vi "XY_plot_gnuplot.vi"(0 "Plot Array":cluster{dbl[], dbl[]}[](array[cluster])=[{[500.0, 500.0, 953.54, 215.0, 270.0, 320.0, 445.0, 525.0, 600.0, 675.0, 750.0, 825.0, 900.0, 960.0, 1010.0, 1060.0], [4.614524, 4.54365, 5.818368, 0.1374656, 0.6662545, 1.465458, 3.619824, 4.848976, 5.887329, 5.940571, 6.152151, 5.717487, 5.600293, 5.40069, 5.154843, 5.121789]}, {[100.0, 150.0, 215.0, 270.0, 320.0, 445.0, 525.0, 600.0, 675.0, 750.0, 825.0, 900.0, 960.0, 1010.0, 1060.0], [0.002314715, -0.00693192, 0.120417, 0.6880509, 1.519176, 3.513709, 5.065183, 6.116033, 6.096773, 5.938465, 5.593788, 5.5597, 5.387002, 5.304077, 4.887903]}] {"?" format="%.2f"; "?" format="%.2f"}, 1 "Job Directory":path=path "/G4_2_HD/Users/paulhayden/Documents/Projects/Westlakes_resolution") -> (2 "Saved Automatically?":bool, 3 "Tex Info String":string="set term epslatex\nset output \"Plot.eps\"\nset xlabel '$Distance~(m)$'\nset ylabel '$DF~(s/m^3)\\times10^6$'\nset samples 1000\nset pointsize 1.00\nset title '$B38~Centreline~Glc$' 0, 0\nset size 0.75,0.9\n\n#set key 450, -2.5833\n unset key\nset label 1 '~~~~~~~~~~~Angle~(deg)~=~0' at -100, -2.58\nset label 2 '~~~~~~~~~~~Height~(m)~=~5' at -100, -3.27\n set xrange [0 : 500] \n# set autoscale x \n set yrange [0.10000 : 7]\n# set autoscale y \n\nplot \"B38_Centreline_Glc.dat\" index 0 using 1:2 axes x1y1 title '$File=B38R~DDD.xls$' with points 1 1, \\\n\"B38_Centreline_Glc.dat\" index 1 using 1:2 axes x1y1 title '$File=B38R~DDD~1.xls$' with points 1 3", 4 "Plot data file":path)   [LabVIEW 2014]
uses:
  Gnuplot_Label.ctl
  gnuplotScriptComponents/gridlines.ctl
  gnuplotScriptComponents/legendProperties.ctl
  gnuplotScriptComponents/legendAppearance.ctl
  gnuplotScriptComponents/alignment.ctl
  gnuplotScriptComponents/at.ctl
  <vilib>/Analysis/baseanly.llb/Mean (DBL).vi
  Results_plotter_Global.vi
  <vilib>/Analysis/NI_AALBase.lvlib
  <vilib>/Analysis/NI_AALPro.lvlib
panel:
  in  "Show Re-Run Gnuplot?":bool
  in  "Tab Control":T1(tab)
  in  "Plot Title":u16(ring) items=["Title String Only", "Project::", "Case2::", "Case::", "Date::", "File::", "Ref Velocity:(m/s):", "Source:Location:X (mm)", "Source:Location:Y (mm)", "Source:Location:Z (mm)", "Source:Internal Diameter:(mm)", "Model:Orientation:", "Carrier:Gas:", "Trace:Gas:", "Q:Source:(l/min)", "Q:Trace:(l/min)", "Source:Density:Ratio", "Source::", "X (mm)::", "Y (mm)::", "Z(mm)::", "Location:XY:", "Location:XZ:", "Profiles::", "U/U(ref)::", "V/U(ref)::", "W/U(ref)::", "u^2/U_{ref}^2::", "v^2/U_{ref}^2::", "w^2/U_{ref}^2::", "uv/U_{ref}^2::", "-uw/U_{ref}^2::", "CU(ref)/Q::(m^{-2})", "c'U(ref)/Q::(m^{-2})", "uc/Q::(m^{-2})", "vc/Q::(m^{-2})", "wc/Q::(m^{-2})", "Measurement:Time:(min)", "U::(m/s)", "U:(m/s):St Error", "V::(m/s)", "W::(m/s)", "W:(m/s):St Error", "u^2::(m/s)^2", "v^2::(m/s)^2", "w^2::(m/s)^2", "uv::(m/s)^2", "uw::(m/s)^2", "C:Trace:(ppm)", "C:Trace (ppm):St Error", "c^2::(ppm)^2", "uc::(ppm m/s)", "vc::(ppm m/s)", "wc::(ppm m/s)", "u^2:(m/s)^2:St Error", "w^2:(m/s)^2:St Error", "U/U(ref)::St Error", "W/U(ref)::St Error", "u^2/U_{ref}^2::St Error", "w^2/U_{ref}^2::St Error", "Raw:Data:Filename", "EnFlo_Tunnel:Inlet_Temp:St Deviation", "Instrumentation::", "Number of:FFID Samples:per Block", "Total Number:of FFID Spikes:Removed", "LDA (U):Timescale Estimate:Integrated to 25%", "Number Of:Measurement:Blocks", "LDA:Sampling Rate:(Hz)", "Number of:LDA Samples:per Block", "Multi Run:Start Time:", "Bkgnd:FF (C):", "Bkgnd Variance:FF (C):", "Seconds:since:1st Jan", "Drift%::", "CU/Q::Err", "EnFlo Lab:labstrat1:Delta T", "GMU:Carrier 2:Gas", "Emission:Velocity:m/s", "Emission:Ratio:", "FF (C):Standard Error:in Variance", "GMU:Source:Type", "Aero_Tunnel:Speed:Meas Velocity", "Multi Run:Row:Number", "EnFlo_Tunnel:FFID:Temp", "FF (C):Calibration:Filename", "Source2:Enable:", "GMU:Source:Dem Q", "Multi Run:Command:Filename", "Thermistor:Temp:", "University:Outside:Temp", "Spires::", "Run::", "Roughness::", "Dem_Uref::", "Comments::", "X:Tunnel:(mm)", "EnFlo_Tunnel:Trav Origin:X Offset", "Run_::", "EnFlo_Tunnel Metadata:Source:Number", "EnFlo_Tunnel Metadata:Model:Trees", "w'::", "EnFlo_Stack:Floor:Surface (mm)", "Z (mm)::Raw", "EnFlo_Tunnel:Shaft:rpm", "u'/U::", "EnFlo_Tunnel:Trav1 Pos:X", "EnFlo_Tunnel:Inlet:K_Factor", "EnFlo_Tunnel:Inlet_Temp:Average", "Number of Measurements"]
  in  "Plot Title":string
  in  "Added labels":i32[](listbox)
  in  "Show Labels?":bool
  in  "Summarise":u16(ring) items=["All Series", "X (mm)=-910__Z(mm)=35__"]
  in  "X Log?":bool
  in  "Y Log?":bool
  in  "Ymin Val":dbl
  in  "Ymin":bool=TRUE
  in  "Xmin Val":dbl
  in  "Xmin":bool=TRUE
  in  "Xmax Val":dbl
  in  "Xmax":bool=TRUE
  in  "Ymax Val":dbl
  in  "Ymax":bool=TRUE
  in  "Major Gridlines":T2
  in  "Minor Gridlines":T2
  out "Time format?":bool
  in  "precision":string
  out "Profile offset":dbl
  in  "Offset?":bool
  in  "Mode":T3
  in  "Separation":dbl=1.2
  in  "Fit Line Width":i32=2
  in  "Fit type":T4(ring)
  in  "Put Coeff\nin Results file":bool
  in  "Analysis":T5(ring)
  in  "Wavelength?":bool
  in  "Auto Zp":bool=TRUE
  in  "Fixed Zp":dbl format="%.2f"
  in  "Something about fit..!":bool
  in  "Fit Line Type":i32=2
  in  "Black and white?":bool
  in  "plot error bars?":bool
  in  "Plot style":u16[](array[ring])=[0, 0, 0, 0, 0, 0, 0, 0, 0, 0, 0] items=["points", "lines", "linespoints"]
  in  "Point Size":dbl=1.2 format="%.2f"
  in  "Graph Height":string="0.9"
  in  "Graph width":string="0.75"
  in  "Show legend?":bool
  in  "Legend Position":u16(ring) items=["LabVIEW calculated", "top left", "top right", "bottom left", "bottom right", "below"]
  in  "Reverse order":bool
  in  "Save data analysis file":bool
  out "Path":path
  in  "Filename Max length":i32=28
  out "With legend":i32=580
  out "No Legend":i32=397
  out "No of Series":i32=2
  out "X location":dbl=-100.0
  out "Y location":dbl=-2.583333333333333
  out "Delta y":dbl=0.6900000000000001
  out "Extra range":dbl
  out "Final Title":string="B38 Centreline Glc"
  out "XY Graph":cluster{dbl[], dbl[]}[](graph)=[{[215.0, 270.0, 320.0, 445.0, 500.0, 500.0, 525.0, 600.0, 675.0, 750.0, 825.0, 900.0, 953.54, 960.0, 1010.0, 1060.0], [0.1374656, 0.6662545, 1.465458, 3.619824, 4.614524, 4.54365, 4.848976, 5.887329, 5.940571, 6.152151, 5.717487, 5.600293, 5.818368, 5.40069, 5.154843, 5.121789]}, {[100.0, 150.0, 215.0, 270.0, 320.0, 445.0, 525.0, 600.0, 675.0, 750.0, 825.0, 900.0, 960.0, 1010.0, 1060.0], [0.002314715, -0.00693192, 0.120417, 0.6880509, 1.519176, 3.513709, 5.065183, 6.116033, 6.096773, 5.938465, 5.593788, 5.5597, 5.387002, 5.304077, 4.887903]}]
  # "Scales"
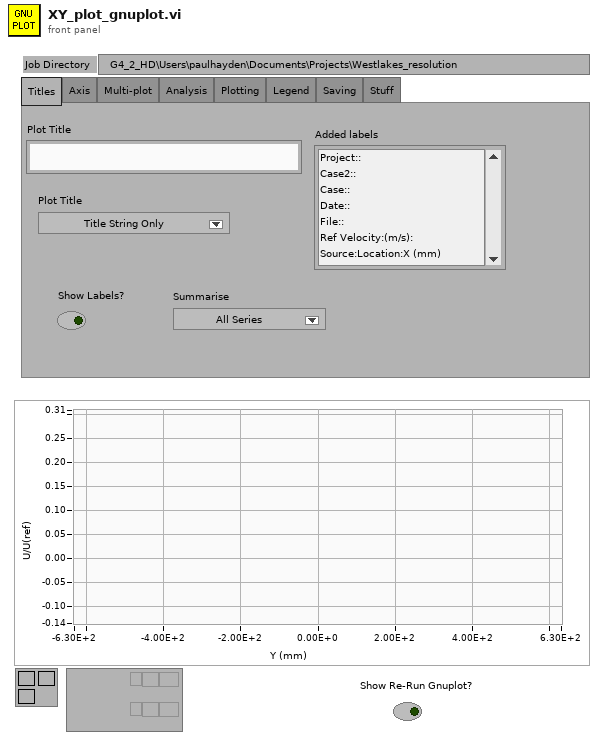
[diagram p1: front panel]
types:
  T1 = enum32{"Titles", "Axis", "Multi-plot", "Analysis", "Plotting", "Legend", "Saving", "Stuff"}
  T2 = typedef "gridlines.ctl" = enum16{"None", "X only", "Y only", "Both X and Y"}
  T3 = typedef "Gnuplot_Label.ctl" = enum16{"3 Labels per plot", "Only Center label", "Only Bottom Label"}
  T4 = enum16{"None", "Spline", "Linear", "2nd Poly", "3rd Poly", "4th Poly", "Gauss Lat", "Gauss vert", "Gauss Vert with 2 sig", "Guass glc"}
  T5 = enum16{"None", "% change", "Spectrum", "Norm Spec"}
  T6 = cluster{"Output":dbl[], "PercentageDifferenceArray":dbl[]}[]
  T7 = cluster{"Output":dbl[], "PercentageDifferenceArray":dbl[]}
  T8 = typedef "legendProperties.ctl" = cluster{"Appearance":T9, "Alignment":T10, "Location":string, "\"At\" location":T11}
  T9 = typedef "legendAppearance.ctl" = cluster{"layout":string, "text-sample order":string, "key order":string, "surroundingBox":string, "MaxRows":u32, "MaxCols":u32, "WidthAdjust":dbl}
  T10 = typedef "alignment.ctl" = cluster{"Horizontal":string, "Vertical":string}
  T11 = typedef "at.ctl" = cluster{"XcoordSys":string, "YcoordSys":string, "Xvalue":dbl, "Yvalue":dbl}
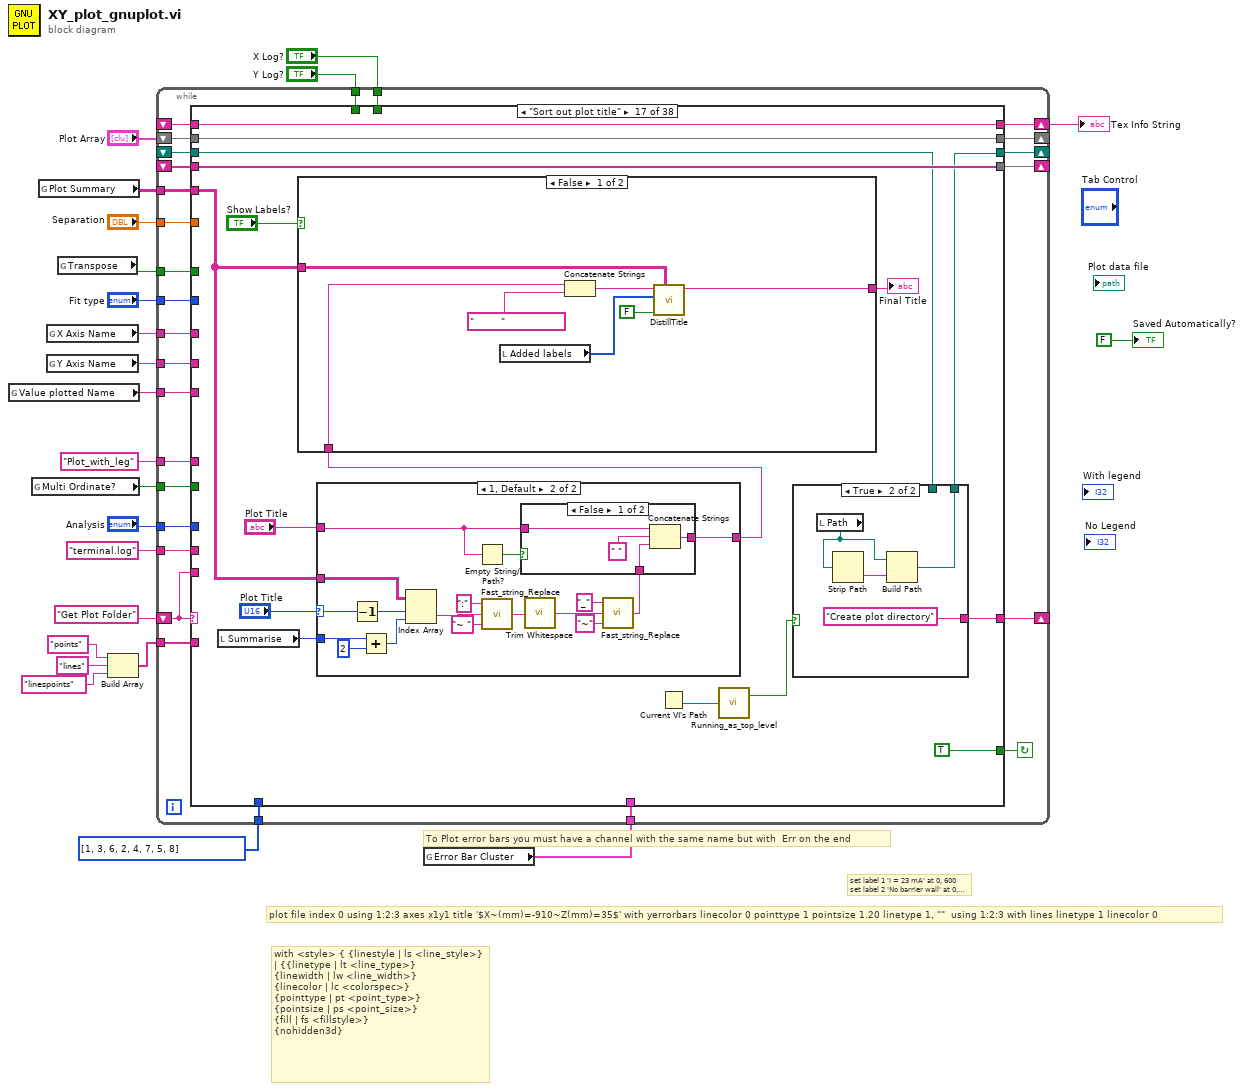
[diagram p0: block diagram]
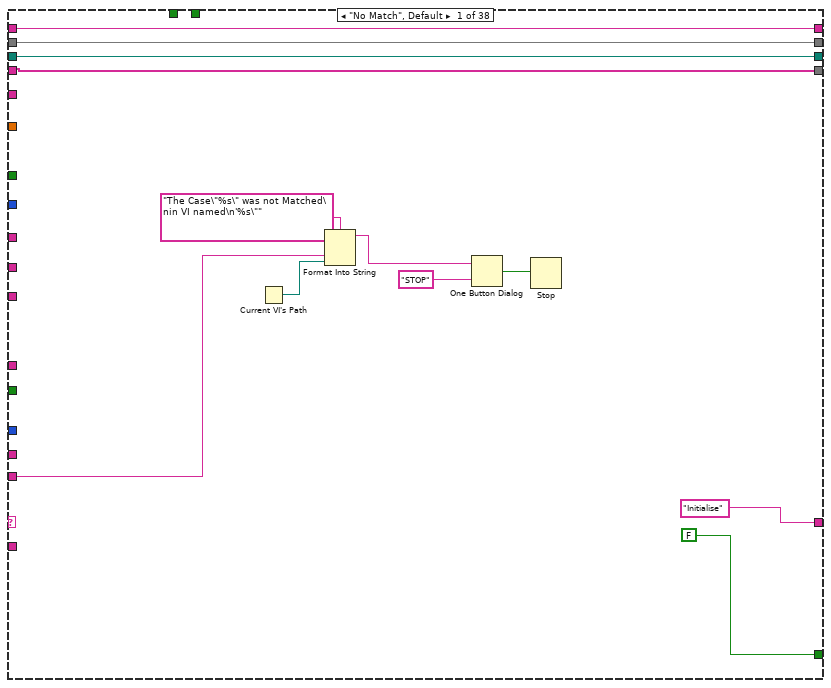
[diagram p2: hidden frame]
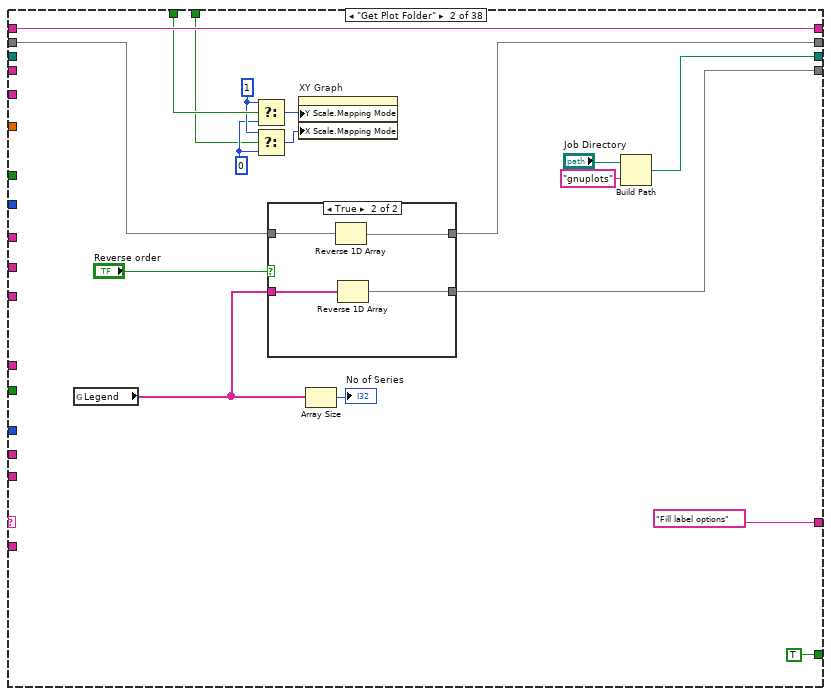
[diagram p3: hidden frame]
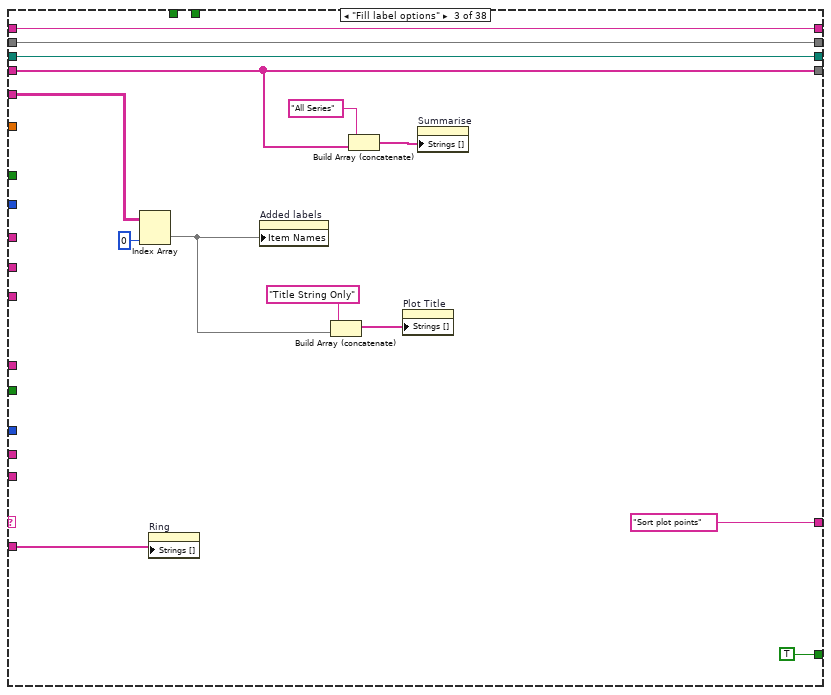
[diagram p5: hidden frame]
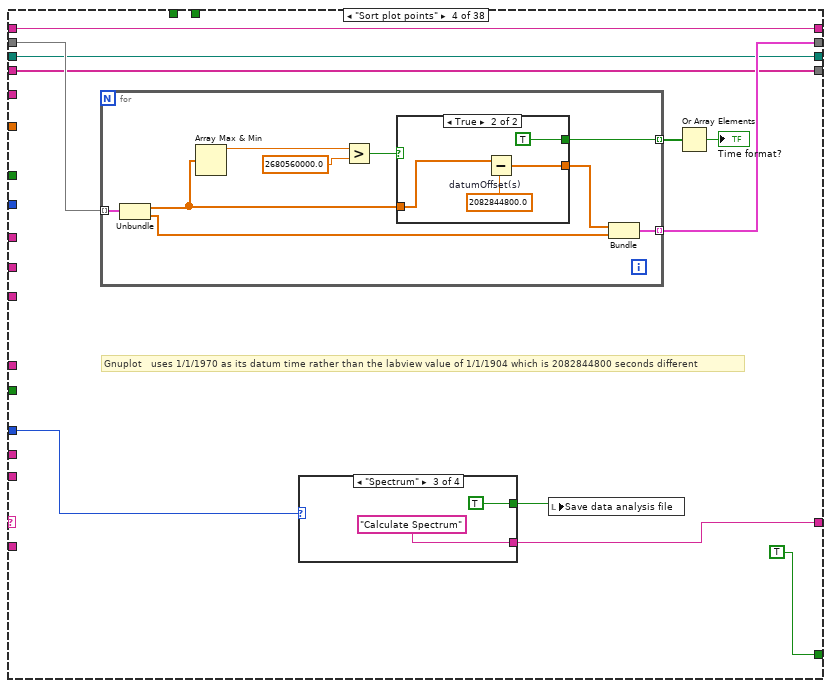
[diagram p6: hidden frame]
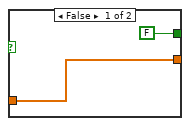
[diagram p7: hidden frame]
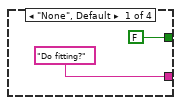
[diagram p8: hidden frame]
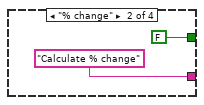
[diagram p9: hidden frame]
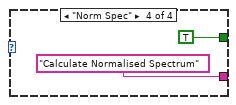
[diagram p10: hidden frame]
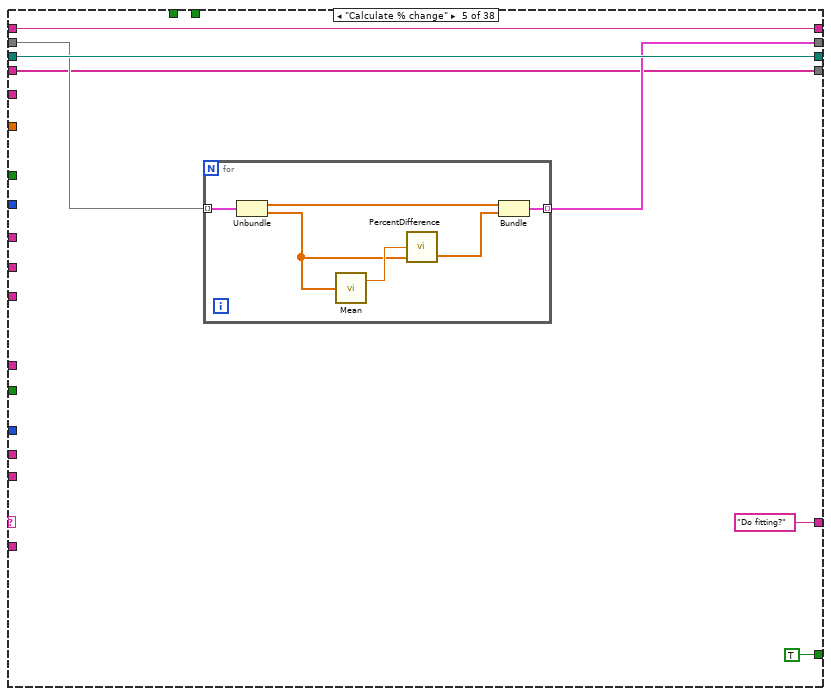
[diagram p11: hidden frame]
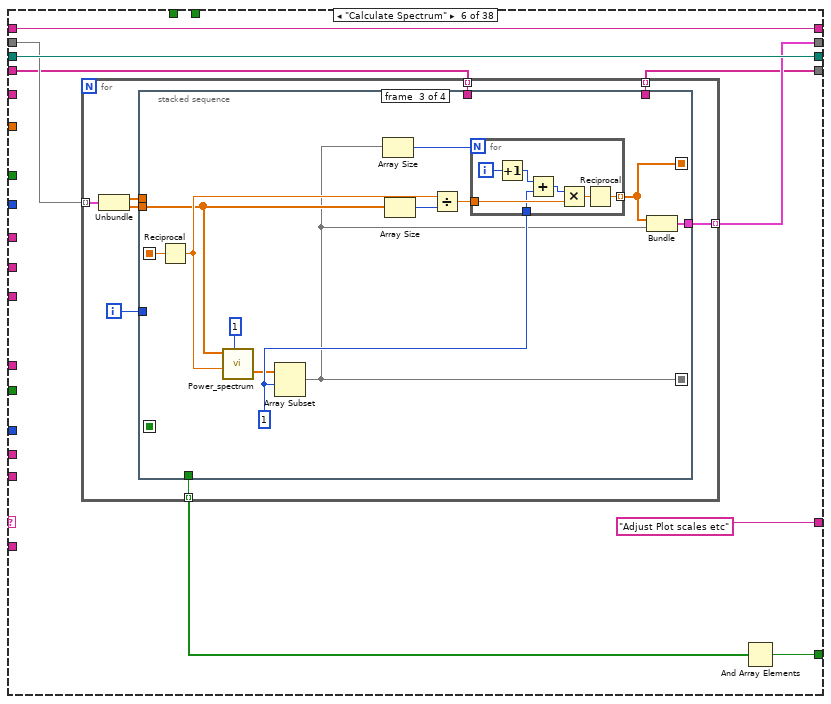
[diagram p12: hidden frame]
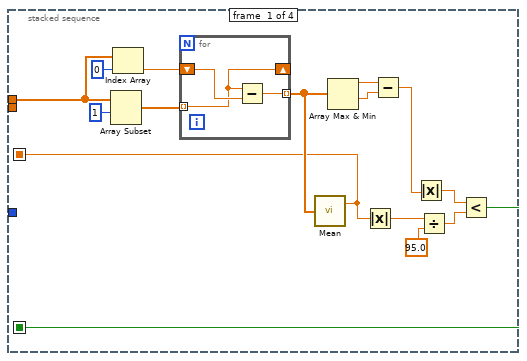
[diagram p13: hidden frame]
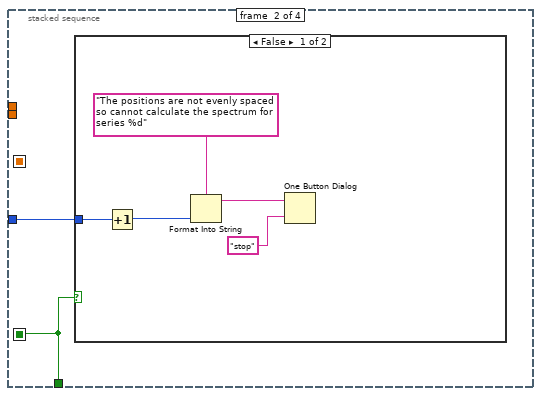
[diagram p14: hidden frame]
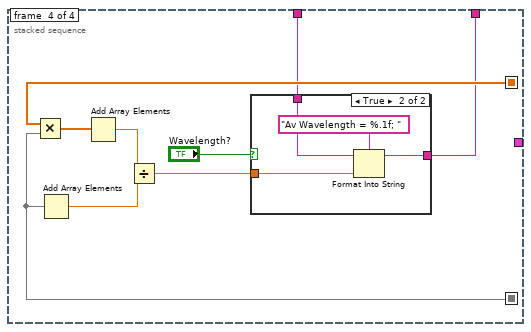
[diagram p16: hidden frame]
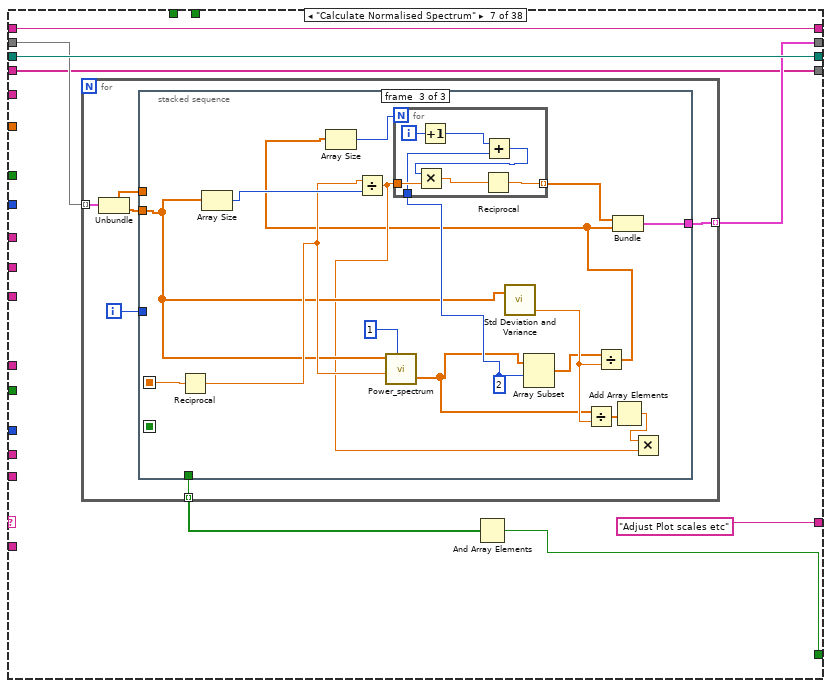
[diagram p18: hidden frame]
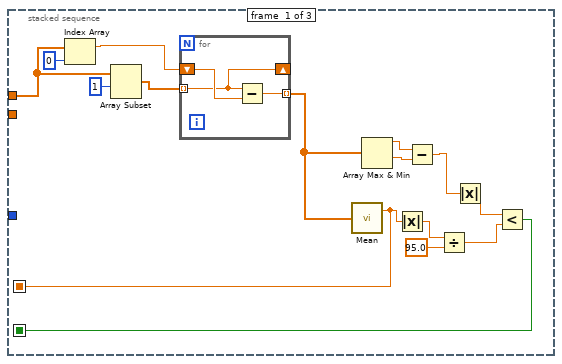
[diagram p19: hidden frame]
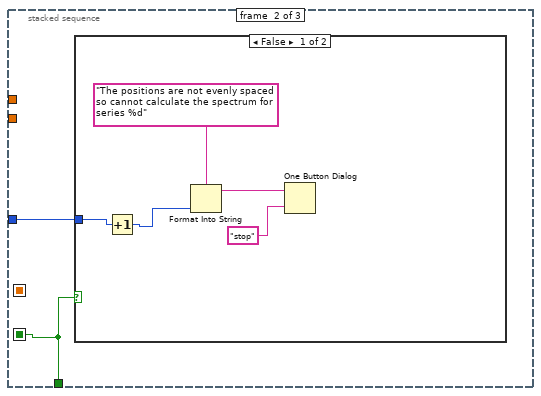
[diagram p20: hidden frame]
diagram:
  # "plot file index 0 using 1:2:3 axes x1y1 title '$X~(mm)=-910~Z(mm)=35$' with yerrorbars linecolor 0 pointtype 1 pointsize 1.20 linetype 1, \"\"  using 1:2:3 with lines linetype 1 linecolor 0"
  # "with <style> { {linestyle | ls <line_style>} \n| {{linetype | lt <line_type>} \n{linewidth | lw <line_width>} \n{linecolor | lc <colorspec>} \n{pointtype | pt <point_type>} \n{pointsize | ps <point_size>} \n{fill | fs <fillstyle>} \n{nohidden3d}"
  # "To Plot error bars you must have a channel with the same name but with  Err on the end"
  # "set label 1 'I = 23 mA' at 0, 600\nset label 2 'No barrier wall' at 0, 300"
  n1 = global read "Results_plotter_Global.vi" "Value plotted Name"() -> (w19:string)
  n2 = global read "Results_plotter_Global.vi" "Multi Ordinate?"() -> (w1:bool)
  n3 = global read "Results_plotter_Global.vi" "Plot Summary"() -> (w22:string[][])
  n4 = global read "Results_plotter_Global.vi" "X Axis Name"() -> (w21:string)
  n5 = global read "Results_plotter_Global.vi" "Y Axis Name"() -> (w20:string)
  n6 = global read "Results_plotter_Global.vi" "Transpose"() -> (w2:bool)
  n7 = Build Array("points", "lines", "linespoints") -> (w9:string[])
  n8 = global read "Results_plotter_Global.vi" "Error Bar Cluster"() -> (w4:cluster{string[]}[])
  n9 = while {
    shift-left: "Get Plot Folder" -> [w48]
    shift-right: [w49] -> _
    tunnel: w22 -> [w47]
    shift-right: [w46] -> _
    shift-left: _ -> [w45]
    tunnel: "Analysis" -> [w44]
    tunnel: w21 -> [w43]
    tunnel: w20 -> [w42]
    tunnel: w19 -> [w41]
    shift-right: [w39] -> _
    shift-left: "Plot Array" -> [w40]
    shift-right: [w37] -> w17
    shift-left: _ -> [w38]
    tunnel: "Plot_with_leg" ("name or relative path") -> [w36]
    tunnel: "Fit type" -> [w35]
    shift-right: [w34] -> _
    shift-left: _ -> [w33]
    tunnel: "terminal.log" -> [w32]
    tunnel: w9 -> [w31]
    tunnel: i32[] [1, 3, 6, 2, 4, 7, 5, 8] ("Plot style") -> [w30]
    tunnel: "Separation" -> [w29]
    tunnel: "Y Log?" -> [w28]
    tunnel: w4 -> [w27]
    tunnel: "X Log?" -> [w26]
    tunnel: w2 -> [w25]
    tunnel: w1 -> [w24]
    stop <- w50 continue-if-true
    n10 = case shown="\"Sort out plot title\"" w48 {
      tunnel: [FALSE TRUE TRUE ("Top Level") TRUE TRUE w150 w223 TRUE TRUE TRUE ("Top Level") TRUE ("Top Level") TRUE ("Top Level") TRUE ("Top Level") TRUE ("Top Level") TRUE ("Top Level") TRUE ("Top Level") TRUE ("Top Level") TRUE ("Top Level") TRUE ("Top Level") TRUE ("Top Level") w674 w747 TRUE ("Top Level") TRUE ("Top Level") TRUE ("Top Level") TRUE ("Top Level") TRUE ("Top Level") TRUE ("Top Level") TRUE ("Top Level") TRUE ("Top Level") TRUE ("Top Level") TRUE ("Top Level") TRUE ("Top Level") TRUE ("Top Level") TRUE ("Top Level") w1570 FALSE ("Top Level") FALSE ("Top Level")] -> w50
      tunnel: ["Initialise" "Fill label options" "Sort plot points" w104 "Do fitting?" "Adjust Plot scales etc" "Adjust Plot scales etc" "Adjust Plot scales etc" "Add fitted line styles" "Adjust Plot scales etc" w381 "Fill Second legend" "Fill Second legend" "Fill Second legend" "Calculate plot max and min values" "Sort out plot title" w566 w636 "Create plot directory" w660 w673 w746 w890 "Edit Legend names" w1074 "Labels?" ("t") "Labels?" ("t") w1235 w1246 "Plot Command" "Write gnuplot file" ("t") "Execute shell script" ("t") "Has pdf been generated?" ("t") w1546 "Input Fit Coefficients into results file?" "Read Fit Coefficients" ("t") "End" ("t") "End" ("t")] -> w49
      tunnel: w48 -> [w57 _ _ _ _ _ _ _ _ _ _ _ _ _ _ _ _ _ _ _ _ _ _ _ _ _ _ _ _ _ _ _ _ _ _ _ _ _]
      tunnel: w47 -> [_ _ w100 _ _ _ _ _ _ _ _ _ _ _ _ _ w575 _ _ _ w672 w745 _ _ _ _ _ _ w1245 _ _ _ _ _ _ _ _ _]
      tunnel: [w54 w77 w94 w108 w139 w155 w229 w290 w305 w366 w391 w417 w426 w438 w465 w499 w568 w637 w648 w662 w675 w748 w902 w942 w1089 w1156 w1212 w1242 w1252 w1376 w1408 w1531 w1539 w1552 w1563 w1574 w1592 w1679] -> w46
      tunnel: w45 -> [w54 _ w94 w108 w139 w155 w229 w290 w305 w366 w391 w417 w426 w438 w461 w499 w567 w633 w649 w657 w675 w748 w902 w942 w1089 w1156 w1212 w1242 w1252 w1376 w1408 w1531 w1539 w1552 w1563 w1574 w1592 w1679]
      tunnel: w44 -> [_ _ _ w105 _ _ _ _ _ _ w382 _ _ w432 _ _ _ w624 _ _ w668 w740 w899 _ _ _ _ _ _ _ _ _ _ _ _ _ _ _]
      tunnel: w43 -> [_ _ _ _ _ _ _ _ w296 _ _ w413 w425 _ _ _ _ _ _ _ w671 w744 w897 _ _ _ _ _ _ _ _ _ _ _ _ _ _ _]
      tunnel: w42 -> [_ _ _ _ _ _ _ _ w295 _ _ w412 w424 w437 _ _ _ _ _ _ w670 w743 w898 _ _ _ _ _ _ _ _ _ _ _ _ _ _ _]
      tunnel: w41 -> [_ _ _ _ _ _ _ _ _ _ _ _ _ _ _ _ _ _ _ _ w667 _ _ _ _ _ _ _ _ _ _ _ _ _ _ _ w1586 _]
      tunnel: w40 -> [w53 w72 w95 w110 w138 w154 w228 w286 w301 w365 w380 w416 w423 w436 w464 w496 w581 w635 w652 w665 w666 w742 w903 w929 w1084 w1151 w1208 w1239 w1247 w1377 w1409 w1537 w1544 w1559 w1568 w1578 w1581 w1684]
      tunnel: [w53 w71 w95 w109 w137 w153 w227 w286 w294 w365 w380 w416 w423 w436 w464 w496 w581 w635 w652 w665 w666 w739 w903 w929 w1084 w1151 w1208 w1239 w1247 w1377 w1409 w1537 w1544 w1559 w1568 w1578 w1581 w1684] -> w39
      tunnel: w38 -> [w52 w76 w96 w107 w136 w152 w226 w289 w304 w363 w383 w415 w422 w435 w463 w500 w576 w634 w651 w664 w676 w749 _ w940 w1088 w1122 w1188 w1230 w1249 w1373 w1406 w1526 w1542 w1557 w1566 w1576 w1595 w1682]
      tunnel: [w52 w76 w96 w107 w136 w152 w226 w289 w304 w363 w383 w415 w422 w435 w463 w500 w576 w634 w651 w664 w676 w749 w893 w938 w1088 w1119 w1187 w1229 w1250 w1369 w1405 w1526 w1542 w1557 w1566 w1576 w1595 w1682] -> w37
      tunnel: w36 -> [_ _ _ _ _ _ _ _ _ _ _ _ _ _ _ _ _ _ _ _ _ _ _ _ _ _ _ _ _ _ _ _ _ _ _ _ _ _]
      tunnel: w35 -> [_ _ _ _ _ _ _ w287 w303 _ w385 _ _ _ _ _ _ _ _ _ _ _ w891 w944 _ _ _ _ _ w1342 w1402 _ _ _ _ w1573 w1588 _]
      tunnel: [w51 w70 w92 w106 w135 w148 w225 w288 w298 w362 w387 w414 w421 w434 w462 w498 w580 w632 w650 w663 w669 w741 w901 w945 w1090 w1155 w1211 w1241 w1251 w1363 w1407 w1532 w1543 w1558 w1567 w1577 w1596 w1683] -> w34
      tunnel: w33 -> [w51 _ w92 w106 w135 w149 w225 w288 w299 w362 w387 w414 w421 w434 w462 w498 w580 w632 w650 w663 w669 w741 w901 w945 w1091 w1155 w1211 w1241 w1251 w1363 w1407 w1532 w1543 w1558 w1567 w1577 w1596 w1683]
      tunnel: w32 -> [_ _ _ _ _ _ _ _ _ _ _ _ _ _ _ _ _ _ _ _ _ _ _ _ _ _ _ _ _ _ _ _ w1538 _ _ _ _ w1677]
      tunnel: w31 -> [_ _ w90 _ _ _ _ _ _ _ _ _ _ _ _ _ _ _ _ _ _ _ _ _ _ _ _ _ _ _ _ _ _ _ _ _ _ _]
      tunnel: w30 -> [_ _ _ _ _ _ _ _ _ _ _ _ _ _ _ _ _ _ _ _ _ _ _ _ _ _ _ _ _ _ w1400 w1528 _ _ _ _ _ _]
      tunnel: w29 -> [_ _ _ _ _ _ _ _ _ _ _ _ _ _ _ _ _ _ _ _ _ w738 _ _ w1083 _ _ _ _ w1360 _ _ _ _ _ _ _ _]
      tunnel: w28 -> [_ w69 _ _ _ _ _ _ _ _ _ _ _ _ _ _ _ _ _ _ _ _ _ _ _ w1135 w1199 _ w1244 w1357 _ _ _ _ _ _ _ _]
      tunnel: w27 -> [_ _ _ _ _ _ _ _ _ _ _ _ _ _ _ w469 _ _ _ _ _ w737 _ _ _ _ _ _ _ _ w1399 _ _ _ _ _ _ _]
      tunnel: w26 -> [_ w64 _ _ _ _ _ _ _ _ _ _ _ _ _ _ _ _ _ _ _ _ _ _ _ w1132 _ _ w1243 w1352 _ _ _ _ _ _ _ _]
      tunnel: w25 -> [_ _ _ _ _ _ _ _ _ _ _ _ _ _ _ w467 _ _ _ _ _ w736 _ w930 _ _ _ _ _ w1347 w1396 _ _ _ _ _ _ _]
      tunnel: w24 -> [_ _ _ _ _ _ _ _ _ _ _ _ _ _ _ _ _ _ _ _ _ _ _ _ _ _ _ _ _ _ _ _ _ _ _ _ _ _]
      frame "No Match", Default {
        n11 = Current VI's Path() -> (path=w56:path)
        n12 = Format Into String(format string="The Case\"%s\" was not Matched\nin VI named\n'%s\"" ("Format String"), w57, w56) -> (resulting string=w60:string)  [unwired: 2 in, 1 out]
        n13 = One Button Dialog(message=w60, button name ("OK")="STOP") -> (true=w58:bool)
        n14 = Stop(stop? (T)=w58) -> ()
      }
      frame "Get Plot Folder" {
        w65 = u8 0 ("f")
        w66 = u8 1 ("Y Scale.Mapping Mode")
        n15 = global read "Results_plotter_Global.vi" "Legend"() -> (w63:string[])
        n16 = Select(t=w66, s=w69, f=w65) -> (s? t:f=w68:u8)
        n17 = Select(t=w66, s=w64, f=w65) -> (s? t:f=w67:u8)
        n18 = case shown="True" "Reverse order" {
          tunnel: w72 -> [w82 w86]
          tunnel: [w82 w85] -> w71
          tunnel: w63 -> [w81 w84]
          tunnel: [w81 w83] -> w70
          frame False {
          }
          frame True {
            n19 = Reverse 1D Array(array=w86) -> (reversed array=w85:T6)
            n20 = Reverse 1D Array(array=w84) -> (reversed array=w83:string[])
          }
        }
        n21 = property on="XY Graph" class="XYGraph (strict)"("Y Scale.Mapping Mode"=w68, "X Scale.Mapping Mode"=w67) -> ()  [unwired: 2 in, 2 out]
        n22 = Array Size(array=w63) -> (size(s)=→"No of Series":i32)
        n23 = Build Path(base path="Job Directory", name or relative path="gnuplots") -> (appended path=w77:path)
      }
      frame "Fill label options" {
        n24 = Index Array(array=w100, index (col)=0 ("disabled index (col)")) -> (element=w88:string[])  [unwired: 1 in]
        n25 = property on="Ring" class="Ring (strict)"("Strings []"=w90) -> ()  [unwired: 2 in, 2 out]
        n26 = property on="Added labels" class="LstBox (strict)"("Item Names"=w88) -> ()  [unwired: 2 in, 2 out]
        n27 = Build Array (concatenate)("Title String Only", w88) -> (w87:string[])
        n28 = Build Array (concatenate)("All Series", w92) -> (w93:string[])
        n29 = property on="Plot Title" class="Ring (strict)"("Strings []"=w87) -> ()  [unwired: 2 in, 2 out]
        n30 = property on="Summarise" class="Ring (strict)"("Strings []"=w93) -> ()  [unwired: 2 in, 2 out]
      }
      frame "Sort plot points" {
        # "Gnuplot   uses 1/1/1970 as its datum time rather than the labview value of 1/1/1904 which is 2082844800 seconds different"
        n31 = for {
          tunnel: w110 -> [w119] mode=indexing
          tunnel: [w120] -> w109 mode=indexing
          tunnel: [w112] -> w102 mode=indexing
          n32 = Unbundle(w119) -> ("Output"=w115:dbl[], "PercentageDifferenceArray"=w116:dbl[])
          n33 = Array Max & Min(array=w115) -> (max value=w118:dbl)  [unwired: 3 out]
          n34 = Greater?(x=w118, y=2680560000.0) -> (0:w113:bool)
          n35 = case shown="True" w113 {
            tunnel: w115 -> [w122 w126]
            tunnel: [w122 w124] -> w114
            tunnel: [FALSE TRUE] -> w112
            frame False {
            }
            frame True {
              w125 = 2082844800.0  # datumOffset(s)
              n36 = Subtract(x=w126, y=w125) -> (x-y=w124:dbl[])
            }
          }
          n37 = Bundle("Output"=w114, "PercentageDifferenceArray"=w116) -> (w120:T7)  [unwired: 1 out]
        }
        n38 = case shown="\"Spectrum\"" w105 {
          tunnel: ["Do fitting?" "Calculate % change" "Calculate Spectrum" "Calculate Normalised Spectrum"] -> w104
          tunnel: [FALSE ("Save data analysis file") FALSE ("Save data analysis file") TRUE ("Save data analysis file") TRUE ("Save data analysis file")] -> w103
          frame "None", Default {
          }
          frame "% change" {
          }
          frame "Spectrum" {
          }
          frame "Norm Spec" {
          }
        }
        n39 = local write "Save data analysis file"(w103) -> ()
        n40 = Or Array Elements(Boolean array=w102) -> (logical OR=→"Time format?":bool)
      }
      frame "Calculate % change" {
        n41 = for {
          tunnel: w138 -> [w147] mode=indexing
          tunnel: [w145] -> w137 mode=indexing
          n42 = Unbundle(w147) -> ("Output"=w146:dbl[], "PercentageDifferenceArray"=w143:dbl[])
          n43 = call-poly <vilib>:"Mean.vi"("X"=w143) -> ("mean"=w144:dbl)  [unwired: 1 out]
          n44 = call "PercentDifference.vi"("CompareeArray"=w143, "Basis"=w144) -> ("PercentageDifferenceArray"=w142:dbl[])  [unwired: 1 in, 1 out]
          n45 = Bundle("Output"=w146, "PercentageDifferenceArray"=w142) -> (w145:T7)  [unwired: 1 out]
        }
      }
      frame "Calculate Spectrum" {
        n46 = for {
          tunnel: w154 -> [w163] mode=indexing
          tunnel: [w164] -> w153 mode=indexing
          tunnel: [w159] -> w151 mode=indexing
          tunnel: w149 -> [w158] mode=indexing
          tunnel: [w157] -> w148 mode=indexing
          i -> [w160]
          n47 = Unbundle(w163) -> ("Output"=w161:dbl[], "PercentageDifferenceArray"=w162:dbl[])
          n48 = stacked-sequence {
            seq-local: [w166 _ _ _] -> [_ _ w196 _]
            seq-local: [w165 _ _ _] -> [_ w183 _ _]
            seq-local: [_ _ w191 _] -> [_ _ _ w216]
            seq-local: [_ _ w190 _] -> [_ _ _ w217]
            tunnel: [_ _ w201 _] -> w164
            tunnel: w162 -> [_ _ w194 _]
            tunnel: w161 -> [w177 _ _ _]
            tunnel: w160 -> [_ w184 _ _]
            tunnel: [_ w183 _ _] -> w159
            tunnel: w158 -> [_ _ _ w212]
            tunnel: [_ _ _ w210] -> w157
            frame #0 {
              n49 = Array Subset(array=w177, index=1) -> (w175:dbl[])  [unwired: 1 in]
              n50 = Index Array(array=w177, index=0) -> (element=w176:dbl)
              n51 = for {
                shift-right: [w181] -> _
                shift-left: w176 -> [w182]
                tunnel: w175 -> [w181] mode=indexing
                tunnel: [w180] -> w172 mode=indexing
                n52 = Subtract(x=w181, y=w182) -> (x-y=w180:dbl)
              }
              n53 = call-poly <vilib>:"Mean.vi"("X"=w172) -> ("mean"=w166:dbl)  [unwired: 1 out]
              n54 = Array Max & Min(array=w172) -> (max value=w174:dbl, min value=w173:dbl)  [unwired: 2 out]
              n55 = Absolute Value(x=w166) -> (abs(x)=w169:dbl)
              n56 = Subtract(x=w174, y=w173) -> (x-y=w171:dbl)
              n57 = Absolute Value(x=w171) -> (abs(x)=w170:dbl)
              n58 = Divide(x=w169, y=95.0) -> (x/y=w167:dbl)
              n59 = Less?(x=w170, y=w167) -> (x < y?=w165:bool)
            }
            frame #1 {
              n60 = case shown="False" w183 {
                tunnel: w184 -> [w189 _]
                frame False {
                  n61 = Increment(x=w189) -> (x+1=w188:i32)
                  n62 = Format Into String(format string="The positions are not evenly spaced so cannot calculate the spectrum for series %d", w188) -> (resulting string=w186:string)  [unwired: 2 in, 1 out]
                  n63 = One Button Dialog(message=w186, button name ("OK")="stop") -> ()  [unwired: 1 out]
                }
                frame True {
                }
              }
            }
            frame #2 {
              w197 = 1 ("index")
              n64 = Reciprocal(x=w196) -> (1/x=w195:dbl)
              n65 = call "Power_spectrum.vi"("U"=w194, "Sampling frequency"=w195, "Block No"=1) -> ("Spectrum output array"=w193:dbl[])  [unwired: 1 in, 2 out]
              n66 = Array Subset(array=w193, index=w197) -> (w190:dbl[])  [unwired: 1 in]
              n67 = Array Size(array=w190) -> (size(s)=w200:i32)
              n68 = Array Size(array=w194) -> (size(s)=w198:i32)
              n69 = Divide(x=w195, y=w198) -> (x/y=w192:dbl)
              n70 = for {
                N: w200 -> [_]
                tunnel: [w205] -> w191 mode=indexing
                tunnel: w192 -> [w207]
                tunnel: w197 -> [w203]
                i -> [w208]
                n71 = Increment(x=w208) -> (x+1=w204:i32)
                n72 = Add(x=w204, y=w203) -> (x+y=w202:i32)
                n73 = Multiply(x=w202, y=w207) -> (x*y=w206:dbl)
                n74 = Reciprocal(x=w206) -> (1/x=w205:dbl)
              }
              n75 = Bundle(w191, w190) -> (w201:cluster{dbl[], dbl[]})  [unwired: 1 out]
            }
            frame #3 {
              n76 = Multiply(x=w216, y=w217) -> (x*y=w215:dbl[])
              n77 = Add Array Elements(numeric array=w217) -> (sum=w213:dbl)
              n78 = Add Array Elements(numeric array=w215) -> (sum=w214:dbl)
              n79 = Divide(x=w214, y=w213) -> (x/y=w211:dbl)
              n80 = case shown="True" "Wavelength?" {
                tunnel: w212 -> [w218 w222]
                tunnel: w211 -> [_ w221]
                tunnel: [w218 w219] -> w210
                frame False {
                }
                frame True {
                  n81 = Format Into String(format string="Av Wavelength = %.1f; ", initial string=w222, w221) -> (resulting string=w219:string)  [unwired: 1 in, 1 out]
                }
              }
            }
          }
        }
        n82 = And Array Elements(Boolean array=w151) -> (logical AND=w150:bool)
      }
      frame "Calculate Normalised Spectrum" {
        n83 = for {
          tunnel: w228 -> [w235] mode=indexing
          tunnel: [w236] -> w227 mode=indexing
          tunnel: [w231] -> w224 mode=indexing
          i -> [w232]
          n84 = Unbundle(w235) -> ("Output"=w233:dbl[], "PercentageDifferenceArray"=w234:dbl[])
          n85 = stacked-sequence {
            seq-local: [w238 _ _] -> [_ _ w271]
            seq-local: [w237 _ _] -> [_ w255 _]
            tunnel: [_ _ w277] -> w236
            tunnel: w234 -> [_ _ w269]
            tunnel: w233 -> [w249 _ _]
            tunnel: w232 -> [_ w256 _]
            tunnel: [_ w255 _] -> w231
            frame #0 {
              n86 = Index Array(array=w249, index=0) -> (element=w248:dbl)
              n87 = Array Subset(array=w249, index=1) -> (w247:dbl[])  [unwired: 1 in]
              n88 = for {
                shift-right: [w253] -> _
                shift-left: w248 -> [w254]
                tunnel: w247 -> [w253] mode=indexing
                tunnel: [w252] -> w244 mode=indexing
                n89 = Subtract(x=w253, y=w254) -> (x-y=w252:dbl)
              }
              n90 = call-poly <vilib>:"Mean.vi"("X"=w244) -> ("mean"=w238:dbl)  [unwired: 1 out]
              n91 = Array Max & Min(array=w244) -> (max value=w246:dbl, min value=w245:dbl)  [unwired: 2 out]
              n92 = Absolute Value(x=w238) -> (abs(x)=w241:dbl)
              n93 = Subtract(x=w246, y=w245) -> (x-y=w243:dbl)
              n94 = Divide(x=w241, y=95.0) -> (x/y=w239:dbl)
              n95 = Absolute Value(x=w243) -> (abs(x)=w242:dbl)
              n96 = Less?(x=w242, y=w239) -> (x < y?=w237:bool)
            }
            frame #1 {
              n97 = case shown="False" w255 {
                tunnel: w256 -> [w261 _]
                frame False {
                  n98 = Increment(x=w261) -> (x+1=w260:i32)
                  n99 = Format Into String(format string="The positions are not evenly spaced so cannot calculate the spectrum for series %d", w260) -> (resulting string=w258:string)  [unwired: 2 in, 1 out]
                  n100 = One Button Dialog(message=w258, button name ("OK")="stop") -> ()  [unwired: 1 out]
                }
                frame True {
                }
              }
            }
            frame #2 {
              w272 = 2 ("index")
              n101 = Reciprocal(x=w271) -> (1/x=w270:dbl)
              n102 = Array Size(array=w269) -> (size(s)=w273:i32)
              n103 = Divide(x=w270, y=w273) -> (x/y=w264:dbl)
              n104 = call "Power_spectrum.vi"("U"=w269, "Sampling frequency"=w270, "Block No"=1) -> ("Spectrum output array"=w267:dbl[])  [unwired: 1 in, 2 out]
              n105 = call <vilib>:"Std Deviation and Variance.vi"("X"=w269) -> ("variance"=w268:dbl)  [unwired: 1 in, 2 out]
              n106 = Array Subset(array=w267, index=w272) -> (w263:dbl[])  [unwired: 1 in]
              n107 = Divide(x=w267, y=w268) -> (x/y=w266:dbl[])
              n108 = Divide(x=w263, y=w268) -> (x/y=w262:dbl[])
              n109 = Array Size(array=w262) -> (size(s)=w276:i32)
              n110 = for {
                N: w276 -> [_]
                tunnel: [w281] -> w275 mode=indexing
                tunnel: w264 -> [w283]
                tunnel: w272 -> [w279]
                i -> [w284]
                n111 = Increment(x=w284) -> (x+1=w280:i32)
                n112 = Add(x=w280, y=w279) -> (x+y=w278:i32)
                n113 = Multiply(x=w278, y=w283) -> (x*y=w282:dbl)
                n114 = Reciprocal(x=w282) -> (1/x=w281:dbl)
              }
              n115 = Bundle(w275, w262) -> (w277:cluster{dbl[], dbl[]})  [unwired: 1 out]
              n116 = Add Array Elements(numeric array=w266) -> (sum=w265:dbl)
              n117 = Multiply(x=w265, y=w264) -> ()  [unwired: 1 out]
            }
          }
        }
        n118 = And Array Elements(Boolean array=w224) -> (logical AND=w223:bool)
      }
      frame "Do fitting?" {
        n119 = case shown="\"None\"" w287 {
          tunnel: ["Adjust Plot scales etc" "Poly fit to data"] -> _
          frame "None" {
          }
          frame "Linear", Default {
          }
        }
      }
      frame "Poly fit to data" {
        n120 = case shown="\"None\", Default" w303 {
          tunnel: [0 ("polynomial order") 1 ("polynomial order") 2 ("polynomial order") 3 ("polynomial order") 4 ("polynomial order")] -> w302
          frame "None", Default {
          }
          frame "Linear" {
          }
          frame "2nd Poly" {
          }
          frame "3rd Poly" {
          }
          frame "4th Poly" {
          }
        }
        n121 = for {
          tunnel: w301 -> [w325] mode=indexing
          tunnel: [w326] -> w300 mode=indexing
          tunnel: w302 -> [w324]
          tunnel: [w319] -> w297 mode=indexing
          tunnel: w296 -> [w318]
          tunnel: w295 -> [w317]
          w323 = 8  # Enhancement factor
          n122 = Unbundle(w325) -> ("Output"=w316:dbl[], "PercentageDifferenceArray"=w315:dbl[])
          n123 = call <vilib>:"General Polynomial Fit.vi"("Y"=w315, "polynomial order"=w324, "X"=w316) -> ("Polynomial Coefficients"=w313:dbl[])  [unwired: 9 in, 3 out]
          n124 = case shown="False" "Something about fit..!" {
            tunnel: [w329 w344] -> w320
            tunnel: [w340 w345] -> w319
            tunnel: w318 -> [w342 _]
            tunnel: w317 -> [w341 _]
            tunnel: w316 -> [w337 _]
            tunnel: w315 -> [w334 _]
            tunnel: w313 -> [_ w344]
            frame False {
              w336 = 0.99 ("Voltage")
              n125 = Build Array (concatenate)(nan ("Voltage"), w334) -> (w338:dbl[])
              n126 = Build Array (concatenate)(w336, w337) -> (w339:dbl[])
              n127 = call "Curve_Fit_ph.vi"("Values In"=w338, "No of points to fit (3)"=4, "Positions"=w339) -> ("Values Out"=w333:dbl[], "Polynomial Fit Coefficients"=w329:dbl[])  [unwired: 1 in]
              n128 = Index Array(array=w333, index=0) -> (element=w331:dbl)
              n129 = call "Number_2_string.vi"("precision"="2", "number"=w331) -> ("String"=w327:string)
              n130 = Format Into String(format string="When %s=%.2f ; %s=%s", w342, w336, w341, w327) -> (resulting string=w340:string)  [unwired: 2 in, 1 out]
            }
            frame True {
              n131 = for {
                shift-right: [w347] -> w345
                shift-left: "" -> [w348]
                tunnel: w344 -> [w351] mode=indexing
                i -> [w352]
                n132 = call "Number_2_string.vi"("number"=w351) -> ("String"=w349:string)  [unwired: 1 in]
                n133 = case shown="0, Default" w352 {
                  tunnel: [w353] -> w350
                  tunnel: w349 -> [w355]
                  frame 0, Default {
                    n134 = Concatenate Strings(w355, " ") -> (w353:string)
                  }
                }
                n135 = Concatenate Strings(w348, w350) -> (w347:string)
              }
            }
          }
          n136 = call "Enhance_No_of_points.vi"("Enhancement factor"=w323, "Input"=w316) -> ("Output"=w322:dbl[])  [unwired: 3 out]
          n137 = for {
            tunnel: w320 -> [w358]
            tunnel: w322 -> [w357] mode=indexing
            tunnel: [w356] -> w321 mode=indexing
            n138 = call "Polynomial_convert.vi"("Calib constants"=w358, "Voltage"=w357) -> ("Eng Values"=w356:dbl)  [unwired: 4 out]
          }
          n139 = Bundle("Output"=w322, w321) -> (w326:cluster{"Output":dbl[], dbl[]})  [unwired: 1 out]
        }
        n140 = Build Array (concatenate)(w299, w297) -> (w298:string[])
        n141 = Build Array (concatenate)(w301, w300) -> (w294:T6)
        n142 = local write "XY Graph"(w294) -> ()
      }
      frame "Add fitted line styles" {
        n143 = local read "No of Series"() -> (w359:i32)
        n144 = Array Subset(array=w362, index=w359) -> (w361:string[])  [unwired: 1 in]
        n145 = for {
          tunnel: w361 -> [w370] mode=indexing
          tunnel: u8 2 ("Plot.Plot Interpolation") -> [w376]
          tunnel: w359 -> [w372]
          i -> [w373]
          w378 = u32 0
          n146 = Concatenate Strings(w370, "  " ("string")) -> (w368:string)
          n147 = Add(x=w372, y=w373) -> (x+y=w371:i32)
          n148 = Quotient & Remainder(x=w373, y=4) -> (x-y*floor(x/y)=w374:i32)  [unwired: 1 out]
          n149 = property on="XY Graph" class="XYGraph (strict)"("Active Plot"=w371, "Plot.Plot Name"=w368, "Plot.Fill/Point Color"=w378, "Plot.Plot Color"=w378, "Plot.Point Style"=u8 0, "Plot.Line Style"=w374, "Plot.Plot Interpolation"=w376) -> ()  [unwired: 2 in, 2 out]
        }
      }
      frame "Adjust Plot scales etc" {
        w379 = u8[] [6, 1, 11, 2, 5, 13, 15, 10, 12, 14]  # pointStyles
        n150 = Greater Than 0?(x=w385) -> (x > 0?=w384:bool)
        n151 = Array Size(array=w387) -> (size(s)=w392:i32)
        n152 = local read "No of Series"() -> (w386:i32)
        n153 = property on="XY Graph" class="XYGraph (strict)"("Legend:Plots Shown"=w392) -> ()  [unwired: 2 in, 2 out]
        n154 = case shown="\"None\", Default" w382 {
          tunnel: ["Adjust plot scales2" "Show percentage change" ("t") "Set spectra axis" ("t") "Set spectra axis" ("t")] -> w381
          frame "None", Default {
          }
          frame "% change" {
          }
          frame "Spectrum" {
          }
          frame "Norm Spec" {
          }
        }
        n155 = Select(t=u8 2 ("Plot.Plot Interpolation"), s=w384, f=u8 0 ("Plot.Plot Interpolation")) -> (s? t:f=w388:u8)
        n156 = for {
          N: w386 -> [_]
          tunnel: w387 -> [w406] mode=indexing
          tunnel: w379 -> [w410]
          tunnel: w388 -> [w399]
          i -> [w409]
          w411 = u32 0
          n157 = String Length(string=w406) -> (length=w402:i32)
          n158 = Subtract(x=w402, y=2) -> (x-y=w400:i32)
          n159 = String Subset(string=w406, offset (0)=0, length (rest)=w400) -> (substring=w405:string)
          n160 = Concatenate Strings(w405, "  " ("string")) -> (w403:string)
          n161 = Index Array(array=w410, index=w409) -> (element=w408:u8)
          n162 = property on="XY Graph" class="XYGraph (strict)"("Active Plot"=w409, "Plot.Plot Name"=w403, "Plot.Fill/Point Color"=w411, "Plot.Plot Color"=w411, "Plot.Point Style"=w408, "Plot.Line Style"=u8 0, "Plot.Plot Interpolation"=w399) -> ()  [unwired: 2 in, 2 out]
        }
        "XY Graph" <- w380
      }
      frame "Adjust plot scales2" {
        n163 = property on="XY Graph" class="XYGraph (strict)"("X Scale.Name Label.Text"=w413, "Y Scale.Name Label.Text"=w412, "Cursor.Visible"=FALSE) -> ()  [unwired: 2 in, 2 out]
      }
      frame "Show percentage change" {
        n164 = Concatenate Strings(w424, " % Change" ("string")) -> (w427:string)
        n165 = property on="XY Graph" class="XYGraph (strict)"("X Scale.Name Label.Text"=w425, "Y Scale.Name Label.Text"=w427, "Cursor.Visible"=FALSE) -> ()  [unwired: 2 in, 2 out]
      }
      frame "Set spectra axis" {
        n166 = case shown="\"Spectrum\", Default" w432 {
          tunnel: [" Spectral Energy" ("string") " Normalised Spectral Energy" ("string")] -> w440
          frame "Spectrum", Default {
          }
          frame "Norm Spec" {
          }
        }
        n167 = Concatenate Strings(w437, w440) -> (w439:string)
        n168 = property on="XY Graph" class="XYGraph (strict)"("X Scale.Name Label.Text"="Wavelength [mm]", "Y Scale.Name Label.Text"=w439, "Cursor.Visible"=FALSE) -> ()  [unwired: 2 in, 2 out]
      }
      frame "Fill Second legend" {
        n169 = global read "Results_plotter_Global.vi" "Current Data Filenames"() -> (w450:string)
        n170 = call "Fast_string_Replace.vi"("Replace match with:"="_", "Input String"=w450, "regular expression"="[/]") -> ("Output String"=w454:string)  [unwired: 2 out]
        n171 = call "Fast_string_Replace.vi"("Replace match with:"="_", "Input String"=w454, "regular expression"="__") -> ("Output String"=w451:string)  [unwired: 2 out]
        n172 = call "Fast_string_Replace.vi"("Replace match with:"="", "Input String"=w451, "regular expression"=" ") -> ("Output String"=w449:string)  [unwired: 2 out]
        n173 = String Subset(string=w449, offset (0)=0, length (rest)=30 ("length (rest)")) -> (substring=w448:string)
        n174 = Build Path(base path=w461, name or relative path=w448) -> (appended path=w465:path)
      }
      frame "Calculate plot max and min values" {
        n175 = local read "plot error bars?"() -> (w468:bool)
        n176 = for {
          tunnel: w496 -> [w524] mode=indexing
          shift-right: [w521] -> w492
          shift-left: _ -> [w517]
          shift-right: [w520] -> w493
          shift-left: _ -> [w516]
          shift-right: [w519] -> w487
          shift-left: _ -> [w515]
          shift-right: [w518] -> w486
          shift-left: _ -> [w514]
          tunnel: w469 -> [w512]
          tunnel: w468 -> [w513]
          tunnel: w467 -> [w510]
          i -> [w511]
          n177 = Unbundle(w524) -> ("Output"=w523:dbl[], "PercentageDifferenceArray"=w522:dbl[])
          n178 = case shown="True" w513 {
            tunnel: w512 -> [_ w545]
            tunnel: w511 -> [_ w544]
            tunnel: [0.0 w540] -> w505
            frame False {
            }
            frame True {
              n179 = Index Array(array=w545, index=w544) -> (element=w543:cluster{string[]})
              n180 = Unbundle(w543) -> (w542:string[])
              n181 = Fract/Exp String To Number(string=w542) -> (number=w541:dbl[])  [unwired: 4 out]
              n182 = Array Max & Min(array=w541) -> (max value=w540:dbl)  [unwired: 3 out]
            }
          }
          n183 = Array Max & Min(array=w523) -> (max value=w503:dbl, min value=w501:dbl)  [unwired: 2 out]
          n184 = Array Max & Min(array=w522) -> (max value=w509:dbl, min value=w507:dbl)  [unwired: 2 out]
          n185 = case shown="True" w510 {
            tunnel: w509 -> [w531 w538]
            tunnel: [w530 w538] -> w508
            tunnel: w507 -> [w529 w537]
            tunnel: [w528 w537] -> w506
            tunnel: w505 -> [w527 w536]
            tunnel: [w526 w532] -> w504
            tunnel: w503 -> [w526 w535]
            tunnel: [w525 w533] -> w502
            tunnel: w501 -> [w525 w534]
            frame False {
              n186 = Subtract(x=w529, y=w527) -> (x-y=w528:dbl)
              n187 = Add(x=w531, y=w527) -> (x+y=w530:dbl)
            }
            frame True {
              n188 = Add(x=w535, y=w536) -> (x+y=w532:dbl)
              n189 = Subtract(x=w534, y=w536) -> (x-y=w533:dbl)
            }
          }
          n190 = case shown="1, Default" w511 {
            tunnel: [w549 w563] -> w521
            tunnel: w504 -> [w549 w562]
            tunnel: w502 -> [w548 w559]
            tunnel: [w548 w558] -> w520
            tunnel: [w547 w551] -> w519
            tunnel: w508 -> [w547 w554]
            tunnel: [w546 w550] -> w518
            tunnel: w506 -> [w546 w552]
            tunnel: w517 -> [_ w564]
            tunnel: w516 -> [_ w561]
            tunnel: w515 -> [_ w555]
            tunnel: w514 -> [_ w553]
            frame 0 {
            }
            frame 1, Default {
              n191 = Greater?(x=w555, y=w554) -> (0:w556:bool)
              n192 = Greater?(x=w564, y=w562) -> (0:w565:bool)
              n193 = Less?(x=w553, y=w552) -> (x < y?=w557:bool)
              n194 = Less?(x=w561, y=w559) -> (x < y?=w560:bool)
              n195 = Select(t=w555, s=w556, f=w554) -> (s? t:f=w551:dbl)
              n196 = Select(t=w553, s=w557, f=w552) -> (s? t:f=w550:dbl)
              n197 = Select(t=w564, s=w565, f=w562) -> (s? t:f=w563:dbl)
              n198 = Select(t=w561, s=w560, f=w559) -> (s? t:f=w558:dbl)
            }
          }
        }
        n199 = Subtract(x=w492, y=w493) -> (x-y=w494:dbl)
        n200 = Subtract(x=w487, y=w486) -> (x-y=w489:dbl)
        n201 = Multiply(x=w494, y=0.1) -> (x*y=w491:dbl)
        n202 = Multiply(x=w489, y=0.1) -> (x*y=w490:dbl)
        n203 = Add(x=w492, y=w491) -> (x+y=w479:dbl)
        n204 = Subtract(x=w493, y=w491) -> (x-y=w476:dbl)
        n205 = Add(x=w487, y=w490) -> (x+y=w472:dbl)
        n206 = Subtract(x=w486, y=w490) -> (x-y=w481:dbl)
        n207 = Select(t=w479, s="Xmax", f="Xmax Val") -> (s? t:f=w477:dbl)
        n208 = Select(t=w476, s="Xmin", f="Xmin Val") -> (s? t:f=w484:dbl)
        n209 = Select(t=w472, s="Ymax", f="Ymax Val") -> (s? t:f=w470:dbl)
        n210 = Select(t=w481, s="Ymin", f="Ymin Val") -> (s? t:f=w485:dbl)
        n211 = property on="XY Graph" class="XYGraph (strict)"("X Scale.Range:Maximum"=w477, "X Scale.Range:Minimum"=w484, "Y Scale.Range:Maximum"=w470, "Y Scale.Range:Minimum"=w485) -> ()  [unwired: 2 in, 2 out]
      }
      frame "Sort out plot title" {
        n212 = local read "Summarise"() -> (w579:u16)
        n213 = case shown="1, Default" "Plot Title" {
          selector: "Plot Title" -> [_ w597]
          tunnel: [w596 w603] -> w574
          tunnel: "Plot Title" -> [w596 w602]
          tunnel: w575 -> [_ w606]
          tunnel: w579 -> [_ w600]
          frame 0 {
          }
          frame 1, Default {
            n214 = Decrement(x=w597) -> (x-1=w605:u16)
            n215 = Add(x=w600, y=u16 2) -> (x+y=w599:u16)
            n216 = Index Array(array=w606, index (row)=w605, index (col)=w599) -> (element=w609:string)
            n217 = Empty String/Path?(string/path=w602) -> (empty?=w604:bool)
            n218 = call "Fast_string_Replace.vi"("Replace match with:"="~ ", "Input String"=w609, "regular expression"=":") -> ("Output String"=w608:string)  [unwired: 2 out]
            n219 = call <vilib>:"Trim Whitespace.vi"("string"=w608) -> ("trimmed string"=w607:string)  [unwired: 1 in]
            n220 = call "Fast_string_Replace.vi"("Replace match with:"="~", "Input String"=w607, "regular expression"="_") -> ("Output String"=w598:string)  [unwired: 2 out]
            n221 = case shown="False" w604 {
              tunnel: [w615 w618] -> w603
              tunnel: w598 -> [w617 w618]
              tunnel: w602 -> [w616 _]
              frame False {
                n222 = Concatenate Strings(w616, " " ("string"), w617) -> (w615:string)
              }
              frame True {
              }
            }
          }
        }
        n223 = case shown="False" "Show Labels?" {
          tunnel: w575 -> [w591 _]
          tunnel: w574 -> [w594 w595]
          tunnel: [w592 w595] -> w573
          frame False {
            n224 = local read "Added labels"() -> (w593:i32[])
            n225 = Concatenate Strings(w594, "         " ("string")) -> (w590:string)
            n226 = call "DistillTitle.vi"("Plot Summary in"=w591, "Show Channels with range of Values?"=FALSE, "Indices to include in Page Title"=w593, "String in"=w590) -> ("String out"=w592:string)  [unwired: 6 in, 1 out]
          }
          frame True {
          }
        }
        "Final Title" <- w573
        n227 = Current VI's Path() -> (path=w571:path)
        n228 = call "Running_as_top_level.vi"("Vi path name"=w571) -> ("Top Level"=w569:bool)  [unwired: 1 out]
        n229 = case shown="True" w569 {
          tunnel: [w583 w586] -> w568
          tunnel: w567 -> [w583 _]
          tunnel: ["Get Filename" ("t") "Create plot directory"] -> w566
          frame False {
          }
          frame True {
            n230 = local read "Path"() -> (w585:path)
            n231 = Strip Path(path=w585) -> (name=w584:string)  [unwired: 1 out]
            n232 = Build Path(base path=w585, name or relative path=w584) -> (appended path=w586:path)
          }
        }
      }
      frame "Get Filename" {
        n233 = local read "Final Title"() -> (w622:string)
        n234 = case shown="\"% change\"" w624 {
          tunnel: ["" "Per_" "Spec_" "N_Spec_"] -> w623
          frame "None" {
          }
          frame "% change" {
          }
          frame "Spectrum" {
          }
          frame "Norm Spec" {
          }
        }
        n235 = Concatenate Strings(w623, w622) -> (w619:string)
        n236 = String Length(string=w622) -> (length=w621:i32)
        n237 = case shown="0" w621 {
          tunnel: [w639 w640] -> w620
          tunnel: w619 -> [w639 w642]
          frame 0 {
          }
          frame 1, Default {
            n238 = Concatenate Strings(w642, "_") -> (w640:string)
          }
        }
        n239 = call "Auto_filename.vi"("Filename Max length"="Filename Max length", "Prefix"=w620) -> ("Filename"=w626:string)
        n240 = Build Path(base path=w633, name or relative path=w626) -> (appended path=w630:path)
        n241 = File/Directory Info(path=w630) -> (error out=w631:errorcluster)  [unwired: 1 in, 6 out]
        n242 = Build Path(base path=w630, name or relative path=w626) -> (appended path=w637:path)
        n243 = Unbundle By Name(w631) -> ("status"=w629:bool)
        n244 = Select(t="Create plot directory", s=w629, f="Find a unique name") -> (s? t:f=w636:string)
      }
      frame "Find a unique name" {
        n245 = call "FindUniqueName.vi"("Max Length"=27, "PathIn"=w649) -> ("UniquedPath"=w648:path)  [unwired: 9 in]
      }
      frame "Create plot directory" {
        n246 = Strip Path(path=w657) -> (stripped path=→"Path":path)  [unwired: 1 out]
        n247 = call "Create_directory_path.vi"("Path name"=w657) -> ("Path name Out"=w662:path)  [unwired: 1 in, 1 out]
        n248 = Select(t="Save data analysis file", s="Save data analysis file", f="Save .dat file") -> (s? t:f=w660:string)
      }
      frame "Save data analysis file" {
        n249 = stacked-sequence {
          seq-local: [w677 _ _] -> [_ _ w721]
          seq-local: [_ w693 _] -> [_ _ w719]
          tunnel: w675 -> [_ _ w732]
          tunnel: [_ _ TRUE ("Top Level")] -> w674
          tunnel: [_ _ "Save .dat file"] -> w673
          tunnel: w672 -> [w680 w695 _]
          tunnel: w671 -> [_ _ _]
          tunnel: w670 -> [_ _ _]
          tunnel: w666 -> [_ w696 _]
          tunnel: w668 -> [w684 _ _]
          tunnel: w667 -> [w683 _ _]
          frame #0 {
            n250 = case shown="\"Norm Spec\"" w684 {
              tunnel: w683 -> [w687 w691]
              tunnel: [w686 w690] -> w682
              tunnel: ["Wavelength::[mm]" "Wavelength::[mm]"] -> w681
              frame "Spectrum", Default {
                n251 = Concatenate Strings(w687, ":Spectral:Energy") -> (w686:string)
              }
              frame "Norm Spec" {
                n252 = Concatenate Strings(w691, ":Normalised Spectral:Energy") -> (w690:string)
              }
            }
            n253 = Index Array(array=w680, index (col)=0 ("disabled index (col)")) -> (element=w678:string[])  [unwired: 1 in]
            n254 = Build Array (concatenate)(w681, w682, w678) -> (w677:string[])
          }
          frame #1 {
            n255 = for {
              tunnel: w696 -> [w707] mode=indexing
              tunnel: w695 -> [w704]
              shift-right: [w698] -> w693
              shift-left: string[][] [] -> [w697]
              i -> [w702]
              n256 = Unbundle(w707) -> ("Output"=w706:dbl[], "PercentageDifferenceArray"=w705:dbl[])
              n257 = Add(x=3 ("disabled index (col)"), y=w702) -> (x+y=w701:i32)
              n258 = Index Array(array=w704, index (col)=w701) -> (element=w700:string[])  [unwired: 1 in]
              n259 = for {
                tunnel: w706 -> [w713] mode=indexing
                tunnel: w705 -> [w712] mode=indexing
                tunnel: w700 -> [w709]
                tunnel: [w708] -> w699 mode=indexing
                n260 = call "Number_2_string.vi"("number"=w713) -> ("String"=w711:string)  [unwired: 1 in]
                n261 = call "Number_2_string.vi"("number"=w712) -> ("String"=w710:string)  [unwired: 1 in]
                n262 = Build Array (concatenate)(w711, w710, w709) -> (w708:string[])
              }
              n263 = Build Array (concatenate)(w697, w699) -> (w698:string[][])
            }
          }
          frame #2 {
            w728 = FALSE  # Append last row only
            w727 = FALSE  # exists?
            n264 = Strip Path(path=w732) -> (stripped path=w733:path, name=w735:string)
            n265 = Array Size(array=w719) -> (size(s)=w718:i32[])
            n266 = Concatenate Strings(w735, ".xls" ("string")) -> (w734:string)
            n267 = Index Array(array=w718, index=0) -> (element=w716:i32)
            n268 = Build Path(base path=w733, name or relative path=w734) -> (appended path=w722:path)
            n269 = Initialize Array("", w716) -> (w715:string[])
            n270 = Build Array (concatenate)(w715, w719) -> (w720:string[][])
            n271 = Initialize Array("", 10 ("Dimension Size")) -> (w726:string[])
            n272 = call "Asterisk_header.vi"("Channel names"=w726) -> ("Header string"=w723:string)
            n273 = call "Write_Ch_data_file.vi"("Append last row only"=w728, "Header string"=w723, "exists?"=w727, "Channel Values"=w720, "Channel names"=w721, "Filename"=w722) -> ()  [unwired: 2 in, 4 out]
          }
        }
      }
      frame "Save .dat file" {
        n274 = stacked-sequence {
          seq-local: [w750 _ _ _ _] -> [_ _ _ _ w870]
          seq-local: [_ w776 _ _ _] -> [_ _ _ _ w871]
          seq-local: [_ _ _ w809 _] -> [_ _ _ _ w872]
          seq-local: [_ _ w793 _ _] -> [_ _ _ w807 _]
          seq-local: [_ _ w785 _ _] -> [_ _ _ w804 _]
          seq-local: [_ _ w787 _ _] -> [_ _ _ w803 _]
          tunnel: w748 -> [_ _ _ _ w875]
          tunnel: [_ _ _ _ TRUE ("Top Level")] -> w747
          tunnel: [_ _ _ _ "Gnuplot script Start"] -> w746
          tunnel: w745 -> [w755 _ _ _ _]
          tunnel: w744 -> [_ w779 _ _ _]
          tunnel: w743 -> [_ w775 _ _ _]
          tunnel: w742 -> [_ _ _ w811 _]
          tunnel: w741 -> [_ _ _ w808 _]
          tunnel: w740 -> [_ w773 _ _ _]
          tunnel: [_ _ _ w806 _] -> w739
          tunnel: w738 -> [_ _ w791 _ _]
          tunnel: w737 -> [_ _ _ w805 _]
          tunnel: w736 -> [_ _ w788 _ _]
          frame #0 {
            n275 = Array Subset(array=w755, length (col)=3 ("length")) -> (w753:string[][])  [unwired: 3 in]
            n276 = Build Array("Column Name", "Numeric Tolerance", "Range of Values") -> (w759:string[])
            n277 = Build Array (concatenate)(w759, w753) -> (w751:string[][])
            n278 = for {
              shift-right: [w763] -> w750
              shift-left: "" -> [w760]
              tunnel: w751 -> [w764] mode=indexing
              n279 = for {
                shift-right: [w765] -> w762
                shift-left: w760 -> [w772]
                tunnel: w764 -> [w766] mode=indexing
                i -> [w771]
                n280 = Equal To 0?(x=w771) -> (x = 0?=w770:bool)
                n281 = Select(t="#", s=w770, f="\t") -> (s? t:f=w767:string)
                n282 = Concatenate Strings(w772, w767, w766) -> (w765:string)
              }
              n283 = Concatenate Strings(w762, "\n") -> (w763:string)
            }
          }
          frame #1 {
            w777 = "\n"
            n284 = case shown="\"% change\"" w773 {
              tunnel: w775 -> [w781 w783]
              tunnel: [w781 w782] -> w774
              frame "None", Default {
              }
              frame "% change" {
                n285 = Concatenate Strings(w783, " %" ("string")) -> (w782:string)
              }
            }
            n286 = Concatenate Strings(w777, w777, "#" ("string"), w779, "\t", w774, w777, w777) -> (w776:string)
          }
          frame #2 {
            n287 = global read "Results_plotter_Global.vi" "Precision"() -> (w790:string[])
            n288 = global read "Results_plotter_Global.vi" "Absisca"() -> (w789:i32)
            n289 = case shown="True" "Offset?" {
              tunnel: [0.0 w801] -> w794
              frame False {
              }
              frame True {
                n290 = property on="XY Graph" class="XYGraph (strict)"() -> ("Y Scale.Range:Maximum"=w800:dbl, "Y Scale.Range:Minimum"=w802:dbl)  [unwired: 2 in, 2 out]
                n291 = Subtract(x=w800, y=w802) -> (x-y=w801:dbl)
              }
            }
            "Profile offset" <- w794
            n292 = Index Array(array=w790, index=w789) -> (element=w786:string)
            n293 = case shown="False" w788 {
              tunnel: ["" w798] -> w787
              tunnel: w786 -> [w795 w798]
              tunnel: [w795 ""] -> w785
              frame False {
              }
              frame True {
              }
            }
            n294 = Multiply(x=w794, y=w791) -> (x*y=w793:dbl)
          }
          frame #3 {
            n295 = for {
              tunnel: w811 -> [w838] mode=indexing
              shift-right: [w837] -> w809
              shift-left: "" -> [w828]
              tunnel: w808 -> [w826] mode=indexing
              tunnel: w807 -> [w823]
              tunnel: [w829] -> w806 mode=indexing
              tunnel: w805 -> [w816] mode=indexing
              tunnel: w804 -> [w813]
              tunnel: w803 -> [w812]
              i -> [w833]
              w836 = "\n"
              n296 = Multiply(x=w823, y=w833) -> (x*y=w818:dbl)
              n297 = Unbundle(w838) -> ("Output"=w831:dbl[], "PercentageDifferenceArray"=w832:dbl[])
              n298 = Negate(x=w818) -> (-x=w817:dbl)
              n299 = call "Number_2_string.vi"("number"=w817) -> ("String"=w825:string)  [unwired: 1 in]
              n300 = Format Into String(format string="\\t%s\\tPlot offset", w825) -> (resulting string=w821:string)  [unwired: 2 in, 1 out]
              n301 = Equal To 0?(x=w818) -> (x = 0?=w822:bool)
              n302 = Select(t="", s=w822, f=w821) -> (s? t:f=w819:string)
              n303 = Unbundle(w816) -> (w815:string[])
              n304 = for {
                tunnel: w831 -> [w857] mode=indexing
                shift-right: [w846] -> w835
                shift-left: "" -> [w847]
                tunnel: w832 -> [w854] mode=indexing
                tunnel: w818 -> [w853]
                tunnel: [w852] -> w830 mode=indexing
                tunnel: w815 -> [w849]
                shift-right: [w845] -> _
                shift-left: string[] [] -> [w844]
                tunnel: w813 -> [w841]
                tunnel: w812 -> [w840]
                i -> [w850]
                w851 = "\t"
                n305 = Subtract(x=w854, y=w853) -> (x-y=w852:dbl)
                n306 = call "Number_2_string.vi"("precision"=w841, "number"=w857) -> ("String"=w856:string)
                n307 = call "Number_2_string.vi"("precision"=w840, "number"=w852) -> ("String"=w855:string)
                n308 = Index Array(array=w849, index=w850) -> (element=w848:string)
                n309 = Concatenate Strings(w856, w851, w855, w851, w848, "\n") -> (w843:string)
                n310 = Search 1D Array(1D array=w844, element=w843) -> (index of element=w842:i32)  [unwired: 1 in]
                n311 = case shown="-1" w842 {
                  tunnel: w847 -> [w859 w864]
                  tunnel: [w859 w863] -> w846
                  tunnel: w843 -> [_ w860]
                  tunnel: w844 -> [w858 w862]
                  tunnel: [w858 w861] -> w845
                  frame 0, Default {
                  }
                  frame -1 {
                    n312 = Concatenate Strings(w864, w860) -> (w863:string)
                    n313 = Build Array (concatenate)(w862, w860) -> (w861:string[])
                  }
                }
              }
              n314 = Bundle("Output"=w831, w830) -> (w829:cluster{"Output":dbl[], dbl[]})  [unwired: 1 out]
              n315 = Concatenate Strings(w828, "#", w826, w819, w836, w835, w836, w836) -> (w837:string)
            }
          }
          frame #4 {
            w867 = FALSE  # advisory dialog? (display:T)
            w868 = FALSE  # append to file? (new file:F)
            n316 = Strip Path(path=w875) -> (stripped path=w876:path, name=w878:string)
            n317 = Concatenate Strings(w870, w871, w872) -> (w869:string)
            n318 = Concatenate Strings(w878, ".dat" ("string")) -> (w877:string)
            n319 = Build Path(base path=w876, name or relative path=w877) -> (appended path=w866:path)
            n320 = call "Write_Characters_To_File.vi"("file path (dialog if empty)"=w866, "advisory dialog? (display:T)"=w867, "character string"=w869, "append to file? (new file:F)"=w868) -> ()  [unwired: 1 in, 4 out]
          }
        }
      }
      frame "Gnuplot script Start" {
        n321 = case shown="\"None\", Default" w899 {
          tunnel: w898 -> [w916 w919 w923 w927]
          tunnel: [w916 w918 w922 w926] -> w886
          tunnel: [w915 w917 "Wavelength [mm]" ("X Axis Name") "Wavelength [mm]" ("X Axis Name")] -> w885
          tunnel: w897 -> [w915 w917 _ _]
          frame "None", Default {
          }
          frame "% change" {
            n322 = Concatenate Strings(w919, " % change" ("string")) -> (w918:string)
          }
          frame "Spectrum" {
            n323 = Concatenate Strings(w923, " Spectral energy" ("string")) -> (w922:string)
          }
          frame "Norm Spec" {
            n324 = Concatenate Strings(w927, " Normalised Spectral Energy" ("string")) -> (w926:string)
          }
        }
        n325 = local read "Final Title"() -> (w887:string)
        n326 = case shown="\"Linear\", Default" w891 {
          tunnel: [w906 w908 "Calculate fit parameters"] -> w890
          tunnel: "Edit Legend names" -> [w906 w908 _]
          tunnel: [w905 w907 "set parametric\nset samples 1000\n"] -> w879
          tunnel: "" -> [w905 w907 _]
          frame "None" {
          }
          frame "Spline" {
          }
          frame "Linear", Default {
          }
        }
        n327 = call "setTerm.vi"() -> ("String out"=w884:string)  [unwired: 10 in, 1 out]
        n328 = call "TypesetInsideMathmode.vi"("DirtyString"=w885) -> ("Mathmode String"=w881:string)  [unwired: 8 in, 2 out]
        n329 = call "TypesetInsideMathmode.vi"("DirtyString"=w886) -> ("Mathmode String"=w880:string)  [unwired: 8 in, 2 out]
        n330 = call "TypesetInsideMathmode.vi"("DirtyString"=w887) -> ("Mathmode String"=w883:string)  [unwired: 8 in, 2 out]
        n331 = local read "Time format?"() -> (w892:bool)
        n332 = call "setTitle.vi"("Title"=w883, "String in"=w884) -> ("String out"=w882:string)  [unwired: 8 in, 1 out]
        n333 = Format Into String(format string="set xlabel '%s'\nset ylabel '%s'\nset size %s,%s\n%s", initial string=w882, w881, w880, "Graph width", "Graph Height", w879) -> (resulting string=w894:string)  [unwired: 1 in, 1 out]
        n334 = case shown="True" w892 {
          tunnel: w894 -> [w911 w913]
          tunnel: [w911 w912] -> w893
          frame False {
          }
          frame True {
            n335 = Concatenate Strings(w913, "\nset xdata time\nset timefmt \"%s\"\nset format  x \"%d %H:%M\"\n") -> (w912:string)
          }
        }
      }
      frame "Calculate fit parameters" {
        # "k=1;    # label 1\nlab=\"23 mA\";\neval( sprintf (\"set label %d %s\", k, lab))"
        n336 = Strip Path(path=w942) -> (name=w941:string)  [unwired: 1 out]
        n337 = Select(t="2:1", s=w930, f="1:2") -> (s? t:f=w931:string)
        n338 = for {
          tunnel: w944 -> [w959]
          tunnel: w941 -> [w957]
          shift-right: [w955] -> w937
          shift-left: w940 -> [w956]
          tunnel: "Auto Zp" -> [w954]
          tunnel: "Fixed Zp" -> [w953]
          tunnel: w931 -> [w952]
          tunnel: w930 -> [w951]
          tunnel: w929 -> [w950] mode=indexing
          i -> [w958]
          n339 = Unbundle(w950) -> ("Output"=w948:dbl[], "PercentageDifferenceArray"=w946:dbl[])
          n340 = case shown="False" w951 {
            tunnel: [w961 w963] -> w949
            tunnel: w948 -> [w961 w962]
            tunnel: [w960 w962] -> w947
            tunnel: w946 -> [w960 w963]
            frame False {
            }
            frame True {
            }
          }
          n341 = case shown="\"Gauss Vert with 2 sig\"" w959 {
            tunnel: w958 -> [w972 w992 w1008 w1027 w1051 w1055 w1061 w1067 _]
            tunnel: w957 -> [w974 w993 w1002 w1032 w1052 w1056 w1062 w1068 _]
            tunnel: w956 -> [w982 w997 w1017 w1042 w1050 w1058 w1064 w1070 w1072]
            tunnel: [w981 w996 w1016 w1041 w1049 w1057 w1063 w1069 w1072] -> w955
            tunnel: w954 -> [_ _ w1007 w1031 _ _ _ _ _]
            tunnel: w953 -> [_ _ w1004 w1028 _ _ _ _ _]
            tunnel: w952 -> [w964 w984 w1001 w1023 w1048 w1054 w1060 w1066 _]
            tunnel: w949 -> [w965 w985 w1000 w1025 _ _ _ _ _]
            tunnel: w947 -> [w966 w986 w999 w1024 _ _ _ _ _]
            frame "Gauss Lat" {
              w969 = 0.01  # A value of zero make gnuplot stop working
              n342 = Array Max & Min(array=w966) -> (max value=w976:dbl, max index (indices)=w973:i32)  [unwired: 2 out]
              n343 = Array Max & Min(array=w965) -> (max value=w980:dbl, min value=w979:dbl)  [unwired: 2 out]
              n344 = Index Array(array=w965, index=w973) -> (element=w968:dbl)
              n345 = Subtract(x=w980, y=w979) -> (x-y=w978:dbl)
              n346 = Divide(x=w978, y=6.0) -> (x/y=w975:dbl)
              n347 = Absolute Value(x=w968) -> (abs(x)=w970:dbl)
              n348 = Greater?(x=w970, y=w969) -> (0:w971:bool)
              n349 = Select(t=w968, s=w971, f=w969) -> (s? t:f=w967:dbl)
              n350 = Format Into String(format string="\nf%d(t) = cmax%d*exp(-((t-offset%d)**2)/(2*sig%d**2))\ncmax%d = %.2f; sig%d = %.2f; offset%d = %.2f           # initial guess for cmax and sig and offset\nfit f%d(t) \"%s.dat\" index %d using %s via cmax%d, sig%d, offset%d #this is a gaussian fit\n", initial string=w982, w972, w972, w972, w972, w972, w976, w972, w975, w972, w967, w972, w974, w972, w964, w972, w972, w972) -> (resulting string=w981:string)  [unwired: 1 in, 1 out]
            }
            frame "Guass glc" {
              w989 = 0.01 ("y")
              n351 = Array Max & Min(array=w986) -> (max value=w995:dbl, max index (indices)=w994:i32)  [unwired: 2 out]
              n352 = Index Array(array=w985, index=w994) -> (element=w988:dbl)
              n353 = Absolute Value(x=w988) -> (abs(x)=w990:dbl)
              n354 = Greater?(x=w990, y=w989) -> (0:w991:bool)
              n355 = Select(t=w988, s=w991, f=w989) -> (s? t:f=w987:dbl)
              n356 = Format Into String(format string="\nf%d(t) = cmax%d*((t/xmax%d)**(-(1+m%d)*q%d)*exp(((1+m%d)/2)*(1-(t/xmax%d)**(-2*q%d))))\ncmax%d = %.2f; xmax%d = %.2f; m%d = 1;  q%d = 0.73         # initial guess for cmax and xmax q and m\nfit f%d(t) \"%s.dat\" index %d using %s via cmax%d, xmax%d, m%d, q%d  #this is a gaussian fit\n", initial string=w997, w992, w992, w992, w992, w992, w992, w992, w992, w992, w995, w992, w987, w992, w992, w992, w993, w992, w984, w992, w992, w992, w992) -> (resulting string=w996:string)  [unwired: 1 in, 1 out]
            }
            frame "Gauss vert" {
              (unwired) "f1(x) = cmax1*exp(-((x-offset1)**2)/(2*sig1**2))"
              n357 = Array Max & Min(array=w999) -> (max value=w1011:dbl, max index (indices)=w1009:i32)  [unwired: 2 out]
              n358 = Array Max & Min(array=w1000) -> (max value=w1015:dbl, min value=w1014:dbl)  [unwired: 2 out]
              n359 = Index Array(array=w1000, index=w1009) -> (element=w1006:dbl)
              n360 = Subtract(x=w1015, y=w1014) -> (x-y=w1013:dbl)
              n361 = Divide(x=w1013, y=6.0) -> (x/y=w1010:dbl)
              n362 = case shown="False" w1007 {
                tunnel: [w1020 w1022] -> w1005
                tunnel: w1006 -> [_ w1022]
                tunnel: w1004 -> [w1020 _]
                tunnel: [w1019 ""] -> w1003
                frame False {
                  w1019 = " #"  # #
                }
                frame True {
                }
              }
              n363 = Format Into String(format string="\nf%d(t) = cmax%d*(exp(-((t-Zp%d)**2)/(2*sigZ%d**2))+exp(-((t+Zp%d)**2)/(2*sigZ%d**2)))\ncmax%d = %.2f; sigZ%d = %.2f; Zp%d = %.2f           # initial guess for cmax and sig and offset\nfit f%d(t) \"%s.dat\" index %d using %s via cmax%d, sigZ%d%s, Zp%d #this is a gaussian fit\n", initial string=w1017, w1008, w1008, w1008, w1008, w1008, w1008, w1008, w1011, w1008, w1010, w1008, w1005, w1008, w1002, w1008, w1001, w1008, w1008, w1003, w1008) -> (resulting string=w1016:string)  [unwired: 1 in, 1 out]
            }
            frame "Gauss Vert with 2 sig" {
              n364 = Array Max & Min(array=w1024) -> (max value=w1034:dbl, max index (indices)=w1036:i32)  [unwired: 2 out]
              n365 = Array Max & Min(array=w1025) -> (max value=w1040:dbl, min value=w1039:dbl)  [unwired: 2 out]
              n366 = Index Array(array=w1025, index=w1036) -> (element=w1030:dbl)
              n367 = Subtract(x=w1040, y=w1039) -> (x-y=w1038:dbl)
              n368 = Divide(x=w1038, y=6.0) -> (x/y=w1033:dbl)
              n369 = call "Vert_Spread_2_Sig.vi"("Index"=w1027) -> ("resulting string"=w1035:string)
              n370 = case shown="False" w1031 {
                tunnel: [w1045 w1047] -> w1029
                tunnel: w1028 -> [w1045 _]
                tunnel: [w1044 ""] -> w1026
                tunnel: w1030 -> [_ w1047]
                frame False {
                  w1044 = " #"  # #
                }
                frame True {
                }
              }
              n371 = Format Into String(format string="\nf%d(t) = %s\ncmax%d = %.2f; sigZ_low%d = %.2f; sigZ_up%d = %.2f; Zp%d = %.2f           # initial guess for cmax and sig and offset\nfit f%d(t) \"%s.dat\" index %d using %s via cmax%d, sigZ_low%d, sigZ_up%d%s, Zp%d #this is a gaussian fit\n", initial string=w1042, w1027, w1035, w1027, w1034, w1027, w1033, w1027, w1033, w1027, w1029, w1027, w1032, w1027, w1023, w1027, w1027, w1027, w1026, w1027) -> (resulting string=w1041:string)  [unwired: 1 in, 1 out]
            }
            frame "2nd Poly" {
              n372 = Format Into String(format string="\nf%d(t) = c%d*t**2 + b%d*t + a%d\n#a%d = 40; b%d = 300; c%d = 1           # initial guess for cmax and sig and offset\nfit f%d(t) \"%s.dat\" index %d using %s via a%d, b%d, c%d #this is a 2nd order poly fit\n", initial string=w1050, w1051, w1051, w1051, w1051, w1051, w1051, w1051, w1051, w1052, w1051, w1048, w1051, w1051, w1051) -> (resulting string=w1049:string)  [unwired: 1 in, 1 out]
            }
            frame "3rd Poly" {
              n373 = Format Into String(format string="\nf%d(t) = d%d*t**3 +c%d*t**2 + b%d*t + a%d\n#a%d = 40; b%d = 300; c%d = 1; d%d = 1         # initial guess for cmax and sig and offset\nfit f%d(t) \"%s.dat\" index %d using %s via a%d, b%d, c%d, d%d #this is a 3rd order poly fit\n", initial string=w1058, w1055, w1055, w1055, w1055, w1055, w1055, w1055, w1055, w1055, w1055, w1056, w1055, w1054, w1055, w1055, w1055, w1055) -> (resulting string=w1057:string)  [unwired: 1 in, 1 out]
            }
            frame "4th Poly" {
              n374 = Format Into String(format string="\nf%d(t) = e%d*t**4 + d%d*t**3 +c%d*t**2 + b%d*t + a%d\n#a%d = 40; b%d = 300; c%d = 1; d%d = 1  e%d = 1       # initial guess for cmax and sig and offset\nfit f%d(t) \"%s.dat\" index %d using %s via a%d, b%d, c%d, d%d, e%d #this is a 3rd order poly fit\n", initial string=w1064, w1061, w1061, w1061, w1061, w1061, w1061, w1061, w1061, w1061, w1061, w1061, w1061, w1062, w1061, w1060, w1061, w1061, w1061, w1061, w1061) -> (resulting string=w1063:string)  [unwired: 1 in, 1 out]
            }
            frame "Linear" {
              n375 = Format Into String(format string="\nf%d(t) = b%d*t + c%d\n#a%d = 40; b%d = 300; c%d = 1           # initial guess for cmax and sig and offset\nfit f%d(t) \"%s.dat\" index %d using %s via b%d, c%d #this is a Linear fit\n", initial string=w1070, w1067, w1067, w1067, w1067, w1067, w1067, w1067, w1068, w1067, w1066, w1067, w1067) -> (resulting string=w1069:string)  [unwired: 1 in, 1 out]
            }
            frame "Spline", Default {
            }
          }
        }
        n376 = Concatenate Strings(w937, "save variables 'Coeff.txt'\n") -> (w938:string)
      }
      frame "Edit Legend names" {
        n377 = local read "Profile offset"() -> (w1081:dbl)
        n378 = for {
          tunnel: w1091 -> [w1106] mode=indexing
          tunnel: [w1105] -> w1090 mode=indexing
          tunnel: [w1104] -> w1086
          i -> [w1104]
          n379 = String Length(string=w1106) -> (length=w1109:i32)
          n380 = Subtract(x=w1109, y=2) -> (x-y=w1107:i32)
          n381 = String Subset(string=w1106, length (rest)=w1107) -> (substring=w1099:string)  [unwired: 1 out]
          n382 = Match Pattern(string=w1099, regular expression="=") -> (before substring=w1098:string, match substring=w1097:string, after substring=w1096:string)  [unwired: 2 out]
          n383 = call "Match_Pat_Case_In.vi"("String to match"="legend", "String"=w1098) -> ("offset past match"=w1101:i32)  [unwired: 1 in, 3 out]
          n384 = Greater Than 0?(x=w1101) -> (x > 0?=w1100:bool)
          n385 = case shown="False" w1100 {
            tunnel: [w1110 w1114] -> w1093
            tunnel: w1096 -> [w1111 w1114]
            tunnel: w1098 -> [w1113 _]
            tunnel: w1097 -> [w1112 _]
            frame False {
              n386 = Concatenate Strings(w1113, w1112, w1111) -> (w1110:string)
            }
            frame True {
            }
          }
          n387 = call "Fast_string_Replace.vi"("Replace match with:"=" ", "Input String"=w1093, "regular expression"="_") -> ("Output String"=w1092:string)  [unwired: 2 out]
          n388 = call "Text_for_latex.vi"("Input String"=w1092) -> ("Output String"=w1105:string)
        }
        n389 = Multiply(x=w1083, y=w1081) -> (x*y=w1085:dbl)
        n390 = Decrement(x=w1083) -> (x-1=w1082:dbl)
        n391 = Multiply(x=w1085, y=w1086) -> (x*y=w1080:dbl)
        n392 = Multiply(x=w1081, y=w1082) -> (x*y=w1079:dbl)
        n393 = Add(x=w1079, y=w1080) -> (x+y=→"Extra range":dbl)
        n394 = Equal To 0?(x="Legend Position") -> (x = 0?=w1076:bool)
        n395 = Select(t="Auto Legend Position", s=w1076, f="Specified Legend Position") -> (s? t:f=w1074:string)
      }
      frame "Auto Legend Position" {
        w1117 = T8 {"Appearance"={"layout"="horizontal", "text-sample order"="", "key order"="", "surroundingBox"="", "MaxRows"=0, "MaxCols"=0, "WidthAdjust"=0.0}, "Alignment"={"Horizontal"="center", "Vertical"="bottom"}, "Location"="", "\"At\" location"={"XcoordSys"="", "YcoordSys"="", "Xvalue"=0.0, "Yvalue"=0.0}}  # LegendProperties
        w1115 = "at"  # Location
        # "Don't know if any of this is really required-  maybe for offset plots.....?"
        n396 = property on="XY Graph" class="XYGraph (strict)"() -> ("X Scale.Range:Maximum"=w1126:dbl, "X Scale.Range:Minimum"=w1125:dbl, "Y Scale.Range:Minimum"=w1129:dbl, "Y Scale.Range:Maximum"=w1127:dbl)  [unwired: 2 in, 2 out]
        n397 = local read "Graph Height"() -> (w1137:string)
        n398 = case shown="True" w1132 {
          tunnel: w1126 -> [w1158 w1162]
          tunnel: w1125 -> [w1157 w1161]
          tunnel: [w1158 w1160] -> w1143
          tunnel: [w1157 w1159] -> w1139
          frame False {
          }
          frame True {
            n399 = Logarithm Base 10(1:w1162) -> (0:w1160:dbl)
            n400 = Logarithm Base 10(1:w1161) -> (0:w1159:dbl)
          }
        }
        n401 = case shown="True" w1135 {
          tunnel: w1127 -> [w1164 w1168]
          tunnel: w1129 -> [w1163 w1167]
          tunnel: [w1164 w1166] -> w1150
          tunnel: [w1163 w1165] -> w1128
          frame False {
          }
          frame True {
            n402 = Logarithm Base 10(1:w1167) -> (0:w1165:dbl)
            n403 = Logarithm Base 10(1:w1168) -> (0:w1166:dbl)
          }
        }
        n404 = local read "Extra range"() -> (w1130:dbl)
        n405 = Fract/Exp String To Number(string=w1137) -> (number=w1136:dbl)  [unwired: 4 out]
        n406 = Subtract(x=w1128, y=w1130) -> (x-y=w1149:dbl)
        n407 = Divide(x=0.35 ("y"), y=w1136) -> (x/y=w1148:dbl)
        n408 = Subtract(x=w1150, y=w1149) -> (x-y=w1146:dbl)
        n409 = Subtract(x=w1143, y=w1139) -> (x-y=w1142:dbl)
        n410 = Multiply(x=w1146, y=w1148) -> (x*y=w1152:dbl)
        n411 = Divide(x=w1146, y=10.0) -> (x/y=w1144:dbl)
        "Delta y" <- w1144
        n412 = Multiply(x=0.9 ("y"), y=w1142) -> (x*y=w1153:dbl)
        n413 = Multiply(x=w1142, y=-0.2 ("x")) -> (x*y=w1140:dbl)
        n414 = Subtract(x=w1149, y=w1152) -> (x-y=w1134:dbl)
        n415 = case shown="True" "Show legend?" {
          tunnel: w1134 -> [w1175 w1181]
          tunnel: [w1175 w1179] -> w1123
          tunnel: w1144 -> [_ w1182]
          frame False {
          }
          frame True {
            n416 = local read "No of Series"() -> (w1178:i32)
            n417 = Add(x=0.65, y=w1178) -> (x+y=w1177:dbl)
            n418 = Multiply(x=w1182, y=w1177) -> (x*y=w1180:dbl)
            n419 = Subtract(x=w1181, y=w1180) -> (x-y=w1179:dbl)
          }
        }
        "Y location" <- w1123
        n420 = Add(x=w1153, y=w1139) -> (x+y=w1133:dbl)
        n421 = Add(x=w1139, y=w1140) -> (x+y=→"X location":dbl)
        n422 = case shown="True" w1132 {
          tunnel: w1133 -> [w1169 w1171]
          tunnel: [w1169 w1170] -> w1121
          frame False {
          }
          frame True {
            n423 = Power Of 10(x=w1171) -> (10^x=w1170:dbl)
          }
        }
        n424 = case shown="True" w1135 {
          tunnel: w1134 -> [w1172 w1174]
          tunnel: [w1172 w1173] -> w1120
          frame False {
          }
          frame True {
            n425 = Power Of 10(x=w1174) -> (10^x=w1173:dbl)
          }
        }
        n426 = Bundle By Name(cluster=w1117, "\"At\" location.Xvalue"=w1121, "\"At\" location.Yvalue"=w1120, "Location"=w1115) -> (w1116:T8)
        n427 = call "setKey.vi"("LegendProperties"=w1116, "Set?"="Show legend?", "String in"=w1122) -> ("String out"=w1119:string)  [unwired: 7 in, 1 out]
      }
      frame "Specified Legend Position" {
        w1185 = T8 {"Appearance"={"layout"="horizontal", "text-sample order"="", "key order"="", "surroundingBox"="", "MaxRows"=0, "MaxCols"=0, "WidthAdjust"=0.0}, "Alignment"={"Horizontal"="center", "Vertical"="bottom"}, "Location"="", "\"At\" location"={"XcoordSys"="", "YcoordSys"="", "Xvalue"=0.0, "Yvalue"=0.0}}  # LegendProperties
        # "Not sure if stuff below is required, to provide \"Y location\"?"
        n428 = property on="XY Graph" class="XYGraph (strict)"() -> ("Y Scale.Range:Minimum"=w1195:dbl, "Y Scale.Range:Maximum"=w1193:dbl)  [unwired: 2 in, 2 out]
        n429 = local read "Graph Height"() -> (w1201:string)
        n430 = case shown="True" w1199 {
          tunnel: w1193 -> [w1214 w1218]
          tunnel: w1195 -> [w1213 w1217]
          tunnel: [w1214 w1216] -> w1207
          tunnel: [w1213 w1215] -> w1194
          frame False {
          }
          frame True {
            n431 = Logarithm Base 10(1:w1218) -> (0:w1216:dbl)
            n432 = Logarithm Base 10(1:w1217) -> (0:w1215:dbl)
          }
        }
        n433 = local read "Extra range"() -> (w1196:dbl)
        n434 = local read "Show legend?"() -> (w1186:bool)
        n435 = Fract/Exp String To Number(string=w1201) -> (number=w1200:dbl)  [unwired: 4 out]
        n436 = Subtract(x=w1194, y=w1196) -> (x-y=w1206:dbl)
        n437 = Divide(x=0.35 ("y"), y=w1200) -> (x/y=w1205:dbl)
        n438 = local read "Legend Position"() -> (w1189:u16)
        n439 = Subtract(x=w1207, y=w1206) -> (x-y=w1204:dbl)
        n440 = property on="Legend Position" class="Ring (strict)"() -> ("Strings []"=w1190:string[])  [unwired: 2 in, 2 out]
        n441 = Multiply(x=w1204, y=w1205) -> (x*y=w1209:dbl)
        n442 = Index Array(array=w1190, index=w1189) -> (element=w1183:string)
        n443 = Divide(x=w1204, y=10.0) -> (x/y=w1202:dbl)
        n444 = Subtract(x=w1206, y=w1209) -> (x-y=w1198:dbl)
        n445 = case shown="True" w1186 {
          tunnel: w1198 -> [w1219 w1225]
          tunnel: [w1219 w1223] -> w1191
          tunnel: w1202 -> [_ w1226]
          frame False {
          }
          frame True {
            n446 = local read "No of Series"() -> (w1222:i32)
            n447 = Add(x=0.65, y=w1222) -> (x+y=w1221:dbl)
            n448 = Multiply(x=w1226, y=w1221) -> (x*y=w1224:dbl)
            n449 = Subtract(x=w1225, y=w1224) -> (x-y=w1223:dbl)
          }
        }
        n450 = Bundle By Name(cluster=w1185, "Location"=w1183) -> (w1184:T8)
        n451 = local write "Y location"(w1191) -> ()
        n452 = call "setKey.vi"("LegendProperties"=w1184, "Set?"=w1186, "String in"=w1188) -> ("String out"=w1187:string)  [unwired: 7 in, 1 out]
      }
      frame "Labels?" {
        n453 = call "setAxisGrids.vi"("Minor Gridlines"="Minor Gridlines", "Major Gridlines"="Major Gridlines", "String in"=w1230) -> ("String out"=w1229:string)  [unwired: 7 in, 1 out]
        n454 = Array Size(array="Added labels") -> (size(s)=w1238:i32)
        n455 = local read "Show Labels?"() -> (w1232:bool)
        n456 = Greater Than 0?(x=w1238) -> (x > 0?=w1234:bool)
        n457 = And(x=w1232, y=w1234) -> (x .and. y?=w1233:bool)
        n458 = Select(t="Add Labels to plot", s=w1233, f="Set plot ranges" ("t")) -> (s? t:f=w1235:string)
      }
      frame "Add Labels to plot" {
        n459 = stacked-sequence {
          seq-local: [w1253 _] -> [_ w1298]
          tunnel: [_ w1299] -> w1250
          tunnel: w1249 -> [_ w1300]
          tunnel: [_ "Set plot ranges" ("t")] -> w1246
          tunnel: w1245 -> [w1256 _]
          tunnel: w1244 -> [_ w1295]
          tunnel: w1243 -> [_ w1293]
          frame #0 {
            n460 = local read "Added labels"() -> (w1258:i32[])
            n461 = Index Array(array=w1256, index (col)=0 ("disabled index (col)")) -> (element=w1257:string[])  [unwired: 1 in]
            n462 = for {
              tunnel: w1258 -> [w1283] mode=indexing
              tunnel: w1257 -> [w1288]
              tunnel: w1256 -> [w1287]
              tunnel: "Summarise" -> [w1286]
              shift-right: [w1274] -> w1253
              shift-left: string[] [] -> [w1275]
              n463 = Add(x=w1286, y=u16 2) -> (x+y=w1284:u16)
              n464 = Index Array(array=w1287, index (col)=w1284) -> (element=w1282:string[])  [unwired: 1 in]
              n465 = Index Array(array=w1288, index=w1283) -> (element=w1279:string)
              n466 = Index Array(array=w1282, index=w1283) -> (element=w1273:string)
              n467 = call "Fast_string_Replace.vi"("Replace match with:"=" ", "Input String"=w1279, "regular expression"=":") -> ("Output String"=w1278:string)  [unwired: 2 out]
              n468 = call <vilib>:"Trim Whitespace.vi"("string"=w1278) -> ("trimmed string"=w1277:string)  [unwired: 1 in]
              n469 = Match Pattern(string=w1273, regular expression="=") -> (offset past match=w1271:i32)  [unwired: 4 out]
              n470 = Less Than 0?(x=w1271) -> (x < 0?=w1270:bool)
              n471 = Select(t="%s = %s" ("format string"), s=w1270, f="%s %s" ("format string")) -> (s? t:f=w1267:string)
              n472 = Format Into String(format string=w1267, w1277, w1273) -> (resulting string=w1260:string)  [unwired: 2 in, 1 out]
              n473 = Match Pattern(string=w1260, regular expression=";") -> (offset past match=w1265:i32)  [unwired: 4 out]
              n474 = Match Pattern(string=w1260, regular expression=" to ") -> (offset past match=w1264:i32)  [unwired: 4 out]
              n475 = Less Than 0?(x=w1265) -> (x < 0?=w1262:bool)
              n476 = Less Than 0?(x=w1264) -> (x < 0?=w1263:bool)
              n477 = And(x=w1262, y=w1263) -> (x .and. y?=w1261:bool)
              n478 = case shown="False" w1261 {
                tunnel: w1275 -> [w1289 w1292]
                tunnel: [w1289 w1290] -> w1274
                tunnel: w1260 -> [_ w1291]
                frame False {
                }
                frame True {
                  n479 = Build Array (concatenate)(w1292, w1291) -> (w1290:string[])
                }
              }
            }
          }
          frame #1 {
            n480 = local read "Show legend?"() -> (w1294:bool)
            n481 = local read "X location"() -> (w1297:dbl)
            n482 = local read "Delta y"() -> (w1296:dbl)
            n483 = for {
              shift-right: [w1321] -> w1299
              shift-left: w1300 -> [w1322]
              tunnel: w1298 -> [w1318] mode=indexing
              tunnel: w1297 -> [w1304]
              tunnel: w1296 -> [w1323]
              tunnel: w1295 -> [w1317]
              tunnel: w1294 -> [w1306]
              tunnel: w1293 -> [w1302]
              i -> [w1324]
              n484 = call "Text_for_latex.vi"("Input String"=w1318) -> ("Output String"=w1312:string)
              n485 = case shown="False" w1302 {
                tunnel: w1304 -> [w1327 w1329]
                tunnel: [w1327 w1328] -> w1303
                frame False {
                }
                frame True {
                  n486 = Power Of 10(x=w1329) -> (10^x=w1328:dbl)
                }
              }
              n487 = String Length(string=w1312) -> (length=w1315:i32)
              n488 = Less?(x=w1315, y=20) -> (x < y?=w1307:bool)
              n489 = Compound Arithmetic op=AND(w1307, invert w1306) -> (w1305:bool)
              n490 = Increment(x=w1324) -> (x+1=w1325:i32)
              n491 = case shown="True" w1305 {
                tunnel: [w1330 w1332] -> w1313
                tunnel: w1312 -> [w1330 w1333]
                tunnel: "~~~~~~~~~~~" -> [_ w1331]
                frame False {
                }
                frame True {
                  n492 = Concatenate Strings(w1331, w1333) -> (w1332:string)
                }
              }
              n493 = Multiply(x=w1324, y=w1323) -> (x*y=w1319:dbl)
              n494 = local read "Y location"() -> (w1320:dbl)
              n495 = call "Number_2_string.vi"("number"=w1303) -> ("String"=w1310:string)  [unwired: 1 in]
              n496 = Subtract(x=w1320, y=w1319) -> (x-y=w1316:dbl)
              n497 = case shown="False" w1317 {
                tunnel: w1316 -> [w1334 w1336]
                tunnel: [w1334 w1335] -> w1309
                frame False {
                }
                frame True {
                  n498 = Power Of 10(x=w1336) -> (10^x=w1335:dbl)
                }
              }
              n499 = call "Number_2_string.vi"("number"=w1309) -> ("String"=w1308:string)  [unwired: 1 in]
              n500 = Format Into String(format string="set label %d '%s' at %s, %s\n", initial string=w1322, w1325, w1313, w1310, w1308) -> (resulting string=w1321:string)  [unwired: 1 in, 1 out]
            }
          }
        }
      }
      frame "Set plot ranges" {
        w1337 = ""
        (unwired) "set border"
        (unwired) "set nologscale  y"
        (unwired) "set logscale  y"
        w1374 = "#"
        w1338 = ""
        n501 = local read "Profile offset"() -> (w1361:dbl)
        n502 = property on="XY Graph" class="XYGraph (strict)"() -> ("X Scale.Range:Maximum"=w1371:dbl, "X Scale.Range:Minimum"=w1370:dbl, "Y Scale.Range:Maximum"=w1354:dbl, "Y Scale.Range:Minimum"=w1355:dbl)  [unwired: 2 in, 2 out]
        n503 = local read "Extra range"() -> (w1365:dbl)
        n504 = Decrement(x=w1360) -> (x-1=w1362:dbl)
        n505 = Multiply(x=w1361, y=w1362) -> (x*y=w1359:dbl)
        n506 = Add(x=w1359, y=w1354) -> (x+y=w1358:dbl)
        n507 = Subtract(x=w1355, y=w1365) -> (x-y=w1366:dbl)
        n508 = call "Number_2_string.vi"("number"=w1358) -> ("String"=w1343:string)  [unwired: 1 in]
        n509 = call "Gnuplot_offset_ytics.vi"("Separation"=w1360, "Mode"="Mode", "precision"="precision", "Legend"=w1363, "Max Plot Value"=w1354, "Profile offset"=w1361) -> ("concatenated string"=w1350:string)
        n510 = call "Number_2_string.vi"("number"=w1371) -> ("String"=w1345:string)  [unwired: 1 in]
        n511 = call "Number_2_string.vi"("number"=w1370) -> ("String"=w1346:string)  [unwired: 1 in]
        n512 = call "Number_2_string.vi"("number"=w1366) -> ("String"=w1344:string)  [unwired: 1 in]
        n513 = case shown="True" w1347 {
          tunnel: [w1384 w1386] -> w1341
          tunnel: w1346 -> [w1384 _]
          tunnel: [w1383 w1385] -> w1340
          tunnel: w1345 -> [w1383 _]
          tunnel: w1344 -> [_ w1386]
          tunnel: w1343 -> [_ w1385]
          frame False {
          }
          frame True {
          }
        }
        n514 = Select(t="\nset logscale  x\n", s=w1352, f=w1338) -> (s? t:f=w1349:string)
        n515 = Select(t="\nset logscale  y\n", s=w1357, f=w1338) -> (s? t:f=w1351:string)
        n516 = case shown="\"Linear\", Default" w1342 {
          tunnel: w1341 -> [_ w1381]
          tunnel: w1340 -> [_ w1380]
          tunnel: ["" w1379] -> w1339
          frame "Spline" {
          }
          frame "Linear", Default {
            n517 = Format Into String(format string="set trange [%s : %s]", w1381, w1380) -> (resulting string=w1379:string)  [unwired: 2 in, 1 out]
          }
        }
        n518 = Format Into String(format string="%s set xrange [%s : %s] \n%s set autoscale x \n%s set yrange [%s : %s]\n%s set autoscale y\n", initial string=w1373, w1337, w1346, w1345, w1374, w1337, w1344, w1343, w1374) -> (resulting string=w1368:string)  [unwired: 1 in, 1 out]
        n519 = Concatenate Strings(w1368, w1339, w1349, w1351, w1350) -> (w1369:string)
      }
      frame "Plot Command" {
        n520 = case shown="True" w1396 {
          tunnel: ["yerrorbars" "xerrorbars"] -> w1395
          tunnel: ["" ", t"] -> w1394
          tunnel: ["t, " ""] -> w1393
          frame False {
          }
          frame True {
          }
        }
        n521 = Strip Path(path=w1408) -> (name=w1390:string)  [unwired: 1 out]
        n522 = Format Into String(format string="\nfile=\"%s.dat\"\n\nplot ", w1390) -> (resulting string=w1391:string)  [unwired: 2 in, 1 out]
        n523 = global read "Results_plotter_Global.vi" "Series Index"() -> (w1397:i32[])
        n524 = for {
          shift-right: [w1454] -> w1389
          shift-left: w1391 -> [w1455]
          tunnel: w1402 -> [w1453]
          tunnel: w1407 -> [w1448] mode=indexing
          tunnel: "Plot style" -> [w1449]
          tunnel: w1400 -> [w1436]
          tunnel: w1399 -> [w1447] mode=indexing
          tunnel: "plot error bars?" -> [w1443]
          tunnel: w1395 -> [w1427]
          tunnel: w1397 -> [w1420] mode=indexing
          tunnel: w1394 -> [w1423]
          tunnel: w1393 -> [w1422]
          tunnel: "Fit Line Width" -> [w1416]
          i -> [w1424]
          n525 = Index Array(array=w1449, index=w1420) -> (element=w1431:u16)
          n526 = Quotient & Remainder(x=w1420, y=8) -> (x-y*floor(x/y)=w1435:i32)  [unwired: 1 out]
          n527 = call "Fast_string_Replace.vi"("Replace match with:"="", "Input String"=w1448, "regular expression"="[$]") -> ("Output String"=w1438:string)  [unwired: 2 out]
          n528 = case shown="2" w1431 {
            tunnel: ["points" ("format string") "lines" ("format string") "linespoints" ("format string")] -> w1428
            frame 0, Default {
            }
            frame 1 {
            }
            frame 2 {
            }
          }
          n529 = case shown="\"Gauss Vert with 2 sig\"" w1453 {
            tunnel: w1424 -> [_ w1466 w1473 w1480 w1487 w1495 w1502 w1509 w1516 w1523]
            tunnel: ["" w1467 w1474 w1481 w1489 w1496 w1503 w1510 w1517 w1524] -> w1452
            tunnel: w1420 -> [_ w1465 w1472 w1478 w1486 w1494 w1501 w1508 w1515 w1522]
            tunnel: "Fit Line Type" -> [_ w1464 w1471 w1479 w1485 w1493 w1500 w1507 w1514 w1521]
            tunnel: w1423 -> [_ _ w1469 w1477 w1483 w1491 w1498 w1505 w1512 w1519]
            tunnel: w1422 -> [_ _ w1470 w1476 w1484 w1492 w1499 w1506 w1513 w1520]
            tunnel: w1416 -> [_ w1463 _ _ _ _ _ _ _ _]
            frame "None", Default {
            }
            frame "Spline" {
              n530 = Format Into String(format string="file index %d using 1:2 axes x1y1 title'' linecolor %d lw %d linetype %d  smooth csplines, ", w1466, w1465, w1463, w1464) -> (resulting string=w1467:string)  [unwired: 2 in, 1 out]
            }
            frame "Gauss Lat" {
              n531 = Format Into String(format string="%s cmax%d*exp(-((t-offset%d)**2)/(2*sig%d**2))%s  linecolor %d linetype %d title '', ", w1470, w1473, w1473, w1473, w1469, w1472, w1471) -> (resulting string=w1474:string)  [unwired: 2 in, 1 out]
            }
            frame "Gauss vert" {
              n532 = Format Into String(format string="%s cmax%d*(exp(-((t-Zp%d)**2)/(2*sigZ%d**2))+exp(-((t+Zp%d)**2)/(2*sigZ%d**2)))%s linecolor %d linetype %d title '', ", w1476, w1480, w1480, w1480, w1480, w1480, w1477, w1478, w1479) -> (resulting string=w1481:string)  [unwired: 2 in, 1 out]
            }
            frame "Gauss Vert with 2 sig" {
              n533 = call "Vert_Spread_2_Sig.vi"("Index"=w1487) -> ("resulting string"=w1488:string)
              n534 = Format Into String(format string="%s %s%s  linecolor %d linetype %d title '', ", w1484, w1488, w1483, w1486, w1485) -> (resulting string=w1489:string)  [unwired: 2 in, 1 out]
            }
            frame "Guass glc" {
              n535 = Format Into String(format string="%s cmax%d*((t/xmax%d)**(-(1+m%d)*q%d)*exp(((1+m%d)/2)*(1-(t/xmax%d)**(-2*q%d))))%s  linecolor %d linetype %d title '', ", w1492, w1495, w1495, w1495, w1495, w1495, w1495, w1495, w1491, w1494, w1493) -> (resulting string=w1496:string)  [unwired: 2 in, 1 out]
            }
            frame "2nd Poly" {
              n536 = Format Into String(format string="%s c%d*t**2 + b%d*t + a%d%s  linecolor %d linetype %d title 'fit%d', ", w1499, w1502, w1502, w1502, w1498, w1501, w1500, w1502) -> (resulting string=w1503:string)  [unwired: 2 in, 1 out]
            }
            frame "3rd Poly" {
              n537 = Format Into String(format string="%s d%d*t**3  + c%d*t**2 + b%d*t + a%d %s linecolor %d linetype %d title 'fit%d', ", w1506, w1509, w1509, w1509, w1509, w1505, w1508, w1507, w1509) -> (resulting string=w1510:string)  [unwired: 2 in, 1 out]
            }
            frame "4th Poly" {
              n538 = Format Into String(format string="%s e%d*t**4 + d%d*t**3  + c%d*t**2 + b%d*t + a%d%s  linecolor %d linetype %d title 'fit%d', ", w1513, w1516, w1516, w1516, w1516, w1516, w1512, w1515, w1514, w1516) -> (resulting string=w1517:string)  [unwired: 2 in, 1 out]
            }
            frame "Linear" {
              n539 = Format Into String(format string="%s b%d*t + c%d%s  linecolor %d linetype %d title 'fit%d', ", w1520, w1523, w1523, w1519, w1522, w1521, w1523) -> (resulting string=w1524:string)  [unwired: 2 in, 1 out]
            }
          }
          n540 = Index Array(array=w1436, index=w1435) -> (element=w1418:i32)
          n541 = case shown="True" "Black and white?" {
            tunnel: w1420 -> [w1457 _]
            tunnel: [w1457 0] -> w1419
            frame False {
            }
            frame True {
            }
          }
          n542 = Unbundle(w1447) -> (w1446:string[])
          n543 = Array Size(array=w1446) -> (size(s)=w1445:i32)
          n544 = Greater Than 0?(x=w1445) -> (x > 0?=w1444:bool)
          n545 = And(x=w1444, y=w1443) -> (x .and. y?=w1429:bool)
          n546 = Select(t=w1427, s=w1429, f=w1428) -> (s? t:f=w1426:string)
          n547 = Select(t=":3", s=w1429, f="") -> (s? t:f=w1439:string)
          n548 = Format Into String(format string="file index %d using 1:2%s axes x1y1 title '$%s$' with ", initial string=w1455, w1424, w1439, w1438) -> (resulting string=w1442:string)  [unwired: 1 in, 1 out]
          n549 = Format Into String(format string=" linecolor %d pointtype %d pointsize %.2f linetype %d, ", initial string=w1426, w1419, w1418, "Point Size", w1418) -> (resulting string=w1430:string)  [unwired: 1 in, 1 out]
          n550 = Concatenate Strings(w1442, w1430, w1452, "\\" ("string"), "\n") -> (w1454:string)
        }
        n551 = call "removeLastContinuation.vi"("String in"=w1389) -> ("String out"=w1388:string)  [unwired: 10 in]
        n552 = Concatenate Strings(w1406, w1388) -> (w1405:string)
      }
      frame "Write gnuplot file" {
        w1534 = FALSE  # append to file? (new file:F)
        w1535 = FALSE  # advisory dialog? (display:T)
        n553 = Strip Path(path=w1531) -> (stripped path=w1527:path)  [unwired: 1 out]
        n554 = Build Path(base path=w1527, name or relative path="gnuplot_script.txt") -> (appended path=w1536:path)
        n555 = call "gnuplot_legend.vi"("Plot style"=w1528, "Legend"=w1532) -> ()  [unwired: 1 out]
        n556 = call "Write_Characters_To_File.vi"("file path (dialog if empty)"=w1536, "advisory dialog? (display:T)"=w1535, "character string"=w1526, "append to file? (new file:F)"=w1534) -> ()  [unwired: 1 in, 4 out]
      }
      frame "Execute shell script" {
        n557 = call "Run_Gnuplot_Script.vi"("logfileName"=w1538, "workingDirectory"=w1539) -> ()
      }
      frame "Has pdf been generated?" {
        n558 = Strip Path(path=w1552) -> (stripped path=w1554:path, name=w1556:string)
        n559 = Concatenate Strings(w1556, ".pdf" ("string")) -> (w1555:string)
        n560 = Build Path(base path=w1554, name or relative path=w1555) -> (appended path=w1551:path)
        n561 = call "Does_file_exist_(simple).vi"("Pathname"=w1551) -> ("exists?"=w1550:bool)
        n562 = case shown="False" w1550 {
          tunnel: ["Open Standard output file" ("f") "Input Fit Coefficients into results file?"] -> w1545
          frame False {
          }
          frame True {
          }
        }
        n563 = Select(t="Show Re-Run Gnuplot?", s="Show Re-Run Gnuplot?", f=w1545) -> (s? t:f=w1546:string)
      }
      frame "Show Re-Run Gnuplot?" {
        n564 = Strip Path(path=w1563) -> (stripped path=w1562:path)  [unwired: 1 out]
        n565 = call "Re_run_Gnuplot.vi"("Plot folder (dialog if empty)"=w1562) -> ()  [unwired: 4 out]
      }
      frame "Input Fit Coefficients into results file?" {
        n566 = Greater?(x=w1573, y=T4."Spline" ("Fit type")) -> (0:w1572:bool)
        n567 = And(x="Put Coeff\nin Results file", y=w1572) -> (x .and. y?=w1570:bool)
      }
      frame "Read Fit Coefficients" {
        n568 = call "Fast_string_Replace.vi"("Replace match with:"="", "Input String"=w1586, "regular expression"=":") -> ("Output String"=w1583:string)  [unwired: 2 out]
        n569 = Strip Path(path=w1592) -> (stripped path=w1590:path)  [unwired: 1 out]
        n570 = Build Path(base path=w1590, name or relative path="Coeff.txt") -> (appended path=w1589:path)
        n571 = call "Read_File_Simple.vi"("Filename"=w1589) -> ("string"=w1587:string)  [unwired: 2 in, 7 out]
        n572 = for {
          tunnel: w1588 -> [w1610]
          tunnel: w1587 -> [w1607]
          tunnel: w1583 -> [w1606]
          tunnel: [w1604] -> w1582
          tunnel: w1581 -> [w1603] mode=indexing
          shift-right: [w1599] -> w1579
          shift-left: string[][] [] -> [w1600]
          i -> [w1609]
          n573 = case shown="\"2nd Poly\"" w1610 {
            tunnel: w1609 -> [_ w1631 w1643 w1647 w1663]
            tunnel: [string[] [] w1627 w1639 w1655 w1669] -> w1608
            tunnel: [string[] [] w1623 w1635 w1652 w1666] -> w1605
            frame "None", Default {
            }
            frame "Gauss Lat" {
              n574 = Format Into String(format string="sig%d", w1631) -> (resulting string=w1629:string)  [unwired: 2 in, 1 out]
              n575 = Format Into String(format string="offset%d", w1631) -> (resulting string=w1628:string)  [unwired: 2 in, 1 out]
              n576 = Format Into String(format string="cmax%d", w1631) -> (resulting string=w1630:string)  [unwired: 2 in, 1 out]
              n577 = Build Array(":Max:Lat", ":Sig Y:", ":Yo:") -> (w1623:string[])
              n578 = Build Array(w1630, w1629, w1628) -> (w1627:string[])
            }
            frame "2nd Poly" {
              n579 = Format Into String(format string="b%d", w1643) -> (resulting string=w1641:string)  [unwired: 2 in, 1 out]
              n580 = Format Into String(format string="c%d", w1643) -> (resulting string=w1640:string)  [unwired: 2 in, 1 out]
              n581 = Format Into String(format string="a%d", w1643) -> (resulting string=w1642:string)  [unwired: 2 in, 1 out]
              n582 = Build Array(":Coeff:A", ":Coeff:B", ":Coeff:C") -> (w1635:string[])
              n583 = Build Array(w1642, w1641, w1640) -> (w1639:string[])
            }
            frame "Gauss Vert with 2 sig" {
              n584 = Format Into String(format string="Zp%d", w1647) -> (resulting string=w1656:string)  [unwired: 2 in, 1 out]
              n585 = Format Into String(format string="cmax%d", w1647) -> (resulting string=w1658:string)  [unwired: 2 in, 1 out]
              n586 = Format Into String(format string="sigZ_low%d", w1647) -> (resulting string=w1648:string)  [unwired: 2 in, 1 out]
              n587 = Format Into String(format string="sigZ_up%d", w1647) -> (resulting string=w1657:string)  [unwired: 2 in, 1 out]
              n588 = Build Array(":Max:Vert", ":Sig Z:Upper", ":Sig Z:Lower", ":Zp:") -> (w1652:string[])
              n589 = Build Array(w1658, w1657, w1648, w1656) -> (w1655:string[])
            }
            frame "Gauss vert" {
              n590 = Format Into String(format string="Zp%d", w1663) -> (resulting string=w1670:string)  [unwired: 2 in, 1 out]
              n591 = Format Into String(format string="cmax%d", w1663) -> (resulting string=w1671:string)  [unwired: 2 in, 1 out]
              n592 = Format Into String(format string="sigZ%d", w1663) -> (resulting string=w1662:string)  [unwired: 2 in, 1 out]
              n593 = Build Array(":Max:Vert", ":Sig Z:Upper", ":Sig Z:Lower", ":Zp:") -> (w1666:string[])
              n594 = Build Array(w1671, w1662, w1662, w1670) -> (w1669:string[])
            }
          }
          n595 = Unbundle(w1603) -> ("Output"=w1597:dbl[])  [unwired: 1 out]
          n596 = for {
            tunnel: w1608 -> [w1620] mode=indexing
            tunnel: w1607 -> [w1617]
            tunnel: [w1615] -> w1602 mode=indexing
            n597 = Concatenate Strings(w1620, " = " ("string")) -> (w1618:string)
            n598 = Match Pattern(string=w1617, regular expression=w1618) -> (after substring=w1616:string)  [unwired: 4 out]
            n599 = call "Split_at_return.vi"("String"=w1616) -> ("before substring"=w1615:string)  [unwired: 1 in, 3 out]
          }
          n600 = for {
            tunnel: w1606 -> [w1614]
            tunnel: w1605 -> [w1613] mode=indexing
            tunnel: [w1612] -> w1604 mode=indexing
            n601 = Concatenate Strings(w1614, w1613) -> (w1612:string)
          }
          n602 = Array Size(array=w1597) -> (size(s)=w1598:i32)
          n603 = for {
            N: w1598 -> [_]
            tunnel: w1602 -> [w1611]
            tunnel: [w1611] -> w1601 mode=indexing
          }
          n604 = Build Array (concatenate)(w1600, w1601) -> (w1599:string[][])
        }
        n605 = global write "Results_plotter_Global.vi" "New Chs In"(w1582) -> ()
        n606 = global write "Results_plotter_Global.vi" "New Values In"(w1579) -> ()
      }
      frame "Open Standard output file" {
        n607 = Strip Path(path=w1679) -> (stripped path=w1676:path)  [unwired: 1 out]
        n608 = Format Into String(format string="open \"%s\"", w1677) -> (resulting string=w1675:string)  [unwired: 2 in, 1 out]
        n609 = call <vilib>:"System Exec.vi"("working directory"=w1676, "command line"=w1675) -> ()  [unwired: 4 in, 6 out]
      }
    }
  }
  "Tex Info String" <- w17
  "Saved Automatically?" <- FALSE
